vi "gums_measureLoopV2.vi"(0 "File Name":path=path "D:/users/test.dat", 1 "SaveDataQuery":bool=TRUE, 2 "Gain Cluster 2":T3={"Vsd"="Gate", "I 2probe 2"="Gate", "Vxy"="Gate", "Vxx"="Gate", "I leak BG"="Gate", "I leak TG"="Gate", "I Gain 1"=1000000.0, "V Gain 1"=1.0, "conversion factor BG"=1.0, "Vin / Vout 1"=1.0, "V Gain 2"=1.0, "Vin / Vout 2"=1.0, "V Gain 3"=1.0, "Vin / Vout 3"=1.0, "I Gain 2"=1000000.0, "I Gain 3"=1000000.0, "V BG"="Gate", "V TG"="Gate", "conversion factor TG"=1.0, "Vin / Vout 4"=1.0, "Vin / Vout 5"=1.0, "Manual Gain 1"=1.0, "Manual Gain 2"=1.0, "Manual Gain 3"=1.0} {"conversion factor TG" items=["1 V/V"=1.0, "4 V/V"=4.0, "15 V/V"=15.0, "30 V/V"=30.0, "45 V/V"=45.0]; "I Gain 3" items=["1"=1.0, "10"=10.0, "100"=100.0, "1K"=1000.0, "10K"=10000.0, "100K"=100000.0, "1M"=1000000.0, "10M"=10000000.0, "100M"=100000000.0, "1G"=1000000000.0]; "I Gain 2" items=["1"=1.0, "10"=10.0, "100"=100.0, "1K"=1000.0, "10K"=10000.0, "100K"=100000.0, "1M"=1000000.0, "10M"=10000000.0, "100M"=100000000.0, "1G"=1000000000.0]; "V Gain 3" items=["1"=1.0, "10"=10.0, "100"=100.0, "1K"=1000.0, "10K"=10000.0]; "V Gain 2" items=["1"=1.0, "10"=10.0, "100"=100.0, "1K"=1000.0, "10K"=10000.0]; "conversion factor BG" items=["1 V/V"=1.0, "4 V/V"=4.0, "15 V/V"=15.0, "30 V/V"=30.0, "45 V/V"=45.0]; "V Gain 1" items=["1"=1.0, "10"=10.0, "100"=100.0, "1K"=1000.0, "10K"=10000.0]; "I Gain 1" items=["1"=1.0, "10"=10.0, "100"=100.0, "1K"=1000.0, "10K"=10000.0, "100K"=100000.0, "1M"=1000000.0, "10M"=10000000.0, "100M"=100000000.0, "1G"=1000000000.0]}, 3 "Refresh Rate [ms]":i32=1000 min=0, 4 "Device Cluster":T4={"K2400 1"="", "K2400_1"=FALSE, "K2400 2"="", "K2400_2"=FALSE, "Lockin1"="", "Lockin1 present"=FALSE, "Lockin2"="", "Lockin2 present"=FALSE, "TIC"="", "Tcontrol"="OFF", "DAC"="", "DAC present"=FALSE, "Bfield query"=FALSE, "Wvlen query"=FALSE, "ITC signal"={"ITC"=0, "Signal"=enum."Sensor 1"}, "DMMX"=[["DMM1", ""]]}) -> ()   [LabVIEW 2011]
uses:
  gumLV8p2/D/Labviewsoft/transport/GUMS/Kelvinox drivers/ITCAPPS - Copie.LLB/ITCSignal.ctl
  gumLV8p2/D/Labviewsoft/transport/GUMS/Kelvinox drivers/ITCAPPS - Copie.LLB/ITCSignals.ctl
  gumLV8p2/D/Labviewsoft/transport/GUMS/Kelvinox drivers/BUSGEN.LLB/OxfordAddress.ctl
  stopButton.vi
  DAC/DACreadglobal.vi
  Tglobalvar.vi
  monochromatorcontrol/perHandlemonochromator.vi
  users/nicolas/PHySpec-SDK-1.0.0/Labview-example/libPhyspec/libPhyspec.lvlib
panel:
  out "refnum raw":refnum<file>
  out "DMM all (V)":dbl[](array[numeric])
  out "DMM Array":dbl[][](array[numeric])
  out "DMMX":string[][](array[string])
  out "DAC 2 V [V]":dbl=1916.0
  out "DAC 2 array":dbl[](array[numeric])
  out "Formula4Array":dbl[](array[numeric]) format="%.2f"
  out "Formula3Array":dbl[](array[numeric]) format="%.2f"
  out "Formula2Array":dbl[](array[numeric]) format="%.2f"
  in  "Formula 4":string
  in  "Formula 3":string
  in  "Formula 2":string
  out "Formula1Array":dbl[](array[numeric]) format="%.2f"
  in  "Formula 1":string
  out "Rxy Array":dbl[](array[numeric])
  out "ITC signal":T1={"ITC"=0, "Signal"=enum."Sensor 1"}
  in  "Fig3 Y scale 2":string(combo)="0"
  in  "Y-Axis 4":string(combo)="Gate"
  in  "X-Axis 4":string(combo)="Gate"
  out "Isd 4":cluster{"Bg":dbl[], "V_4probe":dbl[]}(graph)
  in  "Fig3 Y scale":string(combo)="0"
  in  "Y-Axis 3":string(combo)="Gate"
  in  "X-Axis 3":string(combo)="Gate"
  in  "Fig1 Y scale":string(combo)="0"
  in  "Fig2 Y scale":string(combo)="0"
  out "Fig 2":cluster{"Bg":dbl[], "V_4probe":dbl[]}(graph)
  in  "Y-Axis 1":string(combo)="Gate"
  in  "X-Axis 1":string(combo)="Gate"
  out "R4probe array":dbl[](array[numeric])
  out "R2probe array":dbl[](array[numeric])
  out "Itg array":dbl[](array[numeric])
  out "Ibg array":dbl[](array[numeric])
  out "Vxy array":dbl[](array[numeric])
  out "Vxx array":dbl[](array[numeric])
  out "Isd array":dbl[](array[numeric])
  out "Vsd array":dbl[](array[numeric])
  out "Vtg array":dbl[](array[numeric])
  out "Vbg array":dbl[](array[numeric])
  out "R 4probe [kOhm]":dbl=1916.0
  out "V_topgate [V]":dbl=1916.0
  out "V_backgate [V]":dbl=1916.0
  out "Vxy [V]":dbl=1916.0
  out "Vxx [V]":dbl=1916.0
  out "R 2probe [kOhm]":dbl=1916.0
  out "I Leak TG[nA]":dbl=1916.0
  out "I Leak BG [nA]":dbl=1916.0
  out "I 2probe [nA]":dbl=1916.0
  out "Vsd [V]":dbl=1916.0
  out "signal cluster":T5
  out "SetIntr Cluster":cluster{dbl, dbl, dbl, dbl, dbl, dbl, dbl}
  in  "Sensitivity Lockin2":T6(ring)
  in  "Sensitivity Lockin1":T6(ring)
  out "Wavelength array":dbl[](array[numeric])
  out "Wavelength [nm]":dbl=1916.0
  out "Wvlen query":bool
  out "refnum data":refnum<file>
  in  "Y-Axis 2":string(combo)="Gate"
  in  "X-Axis 2":string(combo)="Gate"
  out "I K2400 01":dbl[](array[numeric])
  out "I K2400 02":dbl[](array[numeric])
  out "DAC 4 array":dbl[](array[numeric])
  out "DAC 3 array":dbl[](array[numeric])
  out "B":dbl[](array[numeric])
  out "Lockin2 X":dbl[](array[numeric])
  out "Lockin2 Y":dbl[](array[numeric])
  out "Lockin1 X":dbl[](array[numeric])
  out "B [T]":dbl=1916.0
  out "T [K]":dbl=1916.0
  out "Bfield query":bool
  out "I K2400_2 [A]":dbl=1916.0
  out "Lockin2 Y [V]":dbl=1916.0
  out "Lockin2 X [V]":dbl=1916.0
  out "DAC 4 V [V]":dbl=1916.0
  out "DAC 3 V [V]":dbl=1916.0
  out "I K2400_1 [A]":dbl=1916.0
  out "Lockin1 Y [V]":dbl=1916.0
  out "Lockin1 X [V]":dbl=1916.0
  out "Lockin1 Ampl [V]":dbl=1916.0
  out "K2400 1 [V]":dbl=1916.0
  out "K2400 2 [V]":dbl=1916.0
  out "DAC 1 V [V]":dbl=1916.0
  out "DAC present":bool
  out "K2400_2":bool
  out "K2400 2":refnum<visa-resource-name>="GPIB0::11::INSTR"
  out "DAC":refnum<visa-resource-name>="GPIB0::11::INSTR"
  out "Tcontrol":string
  out "Lockin2 present":bool
  out "Lockin1 present":bool
  out "K2400_1":bool
  out "TIC":refnum<visa-resource-name>="GPIB0::11::INSTR"
  out "Lockin2":refnum<visa-resource-name>="GPIB0::11::INSTR"
  out "Lockin1":refnum<visa-resource-name>="GPIB0::11::INSTR"
  out "K2400 1":refnum<visa-resource-name>="GPIB0::11::INSTR"
  out "Isd":cluster{"Bg":dbl[], "V_4probe":dbl[]}(graph)
  out "Isd 3":cluster{"Bg":dbl[], "V_4probe":dbl[]}(graph)
  out "stopMainLoop":bool
  out "V K2400_01 array":dbl[](array[numeric])
  out "Lockin1 Y":dbl[](array[numeric])
  out "DAC 1 array":dbl[](array[numeric])
  out "V K2400_02 array":dbl[](array[numeric])
  out "T":dbl[](array[numeric])
  out "Time":dbl[](array[numeric])
  out "Time [s]":dbl=1916.0
  in  "stop":bool
  # "Current run values"
  # "Magnetic Field"
  # "Wavelength"
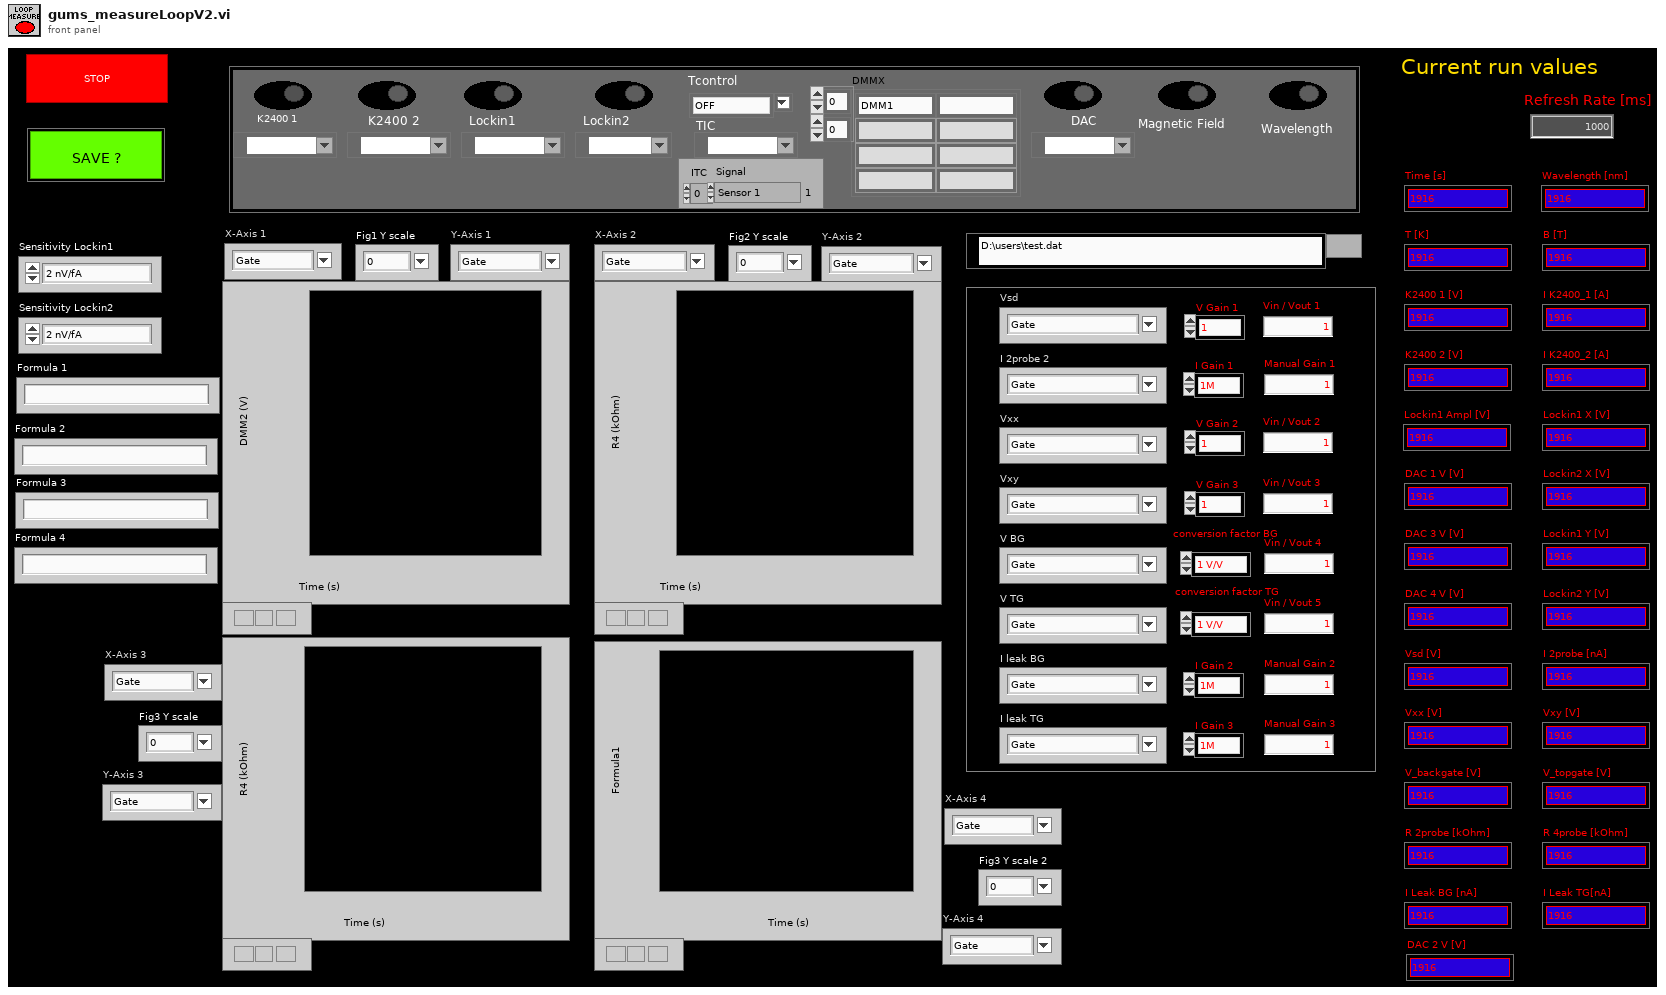
[diagram p1: front panel]
types:
  T1 = typedef "ITCSignal.ctl" = cluster{"ITC":u16, "Signal":T2}
  T2 = typedef "ITCSignals.ctl" = enum16{"Setpoint", "Sensor 1", "Sensor 2", "Sensor 3", "Needle Valve %", "Heater %"}
  T3 = cluster{"Vsd":string, "I 2probe 2":string, "Vxy":string, "Vxx":string, "I leak BG":string, "I leak TG":string, "I Gain 1":dbl, "V Gain 1":dbl, "conversion factor BG":dbl, "Vin / Vout 1":dbl, "V Gain 2":dbl, "Vin / Vout 2":dbl, "V Gain 3":dbl, "Vin / Vout 3":dbl, "I Gain 2":dbl, "I Gain 3":dbl, "V BG":string, "V TG":string, "conversion factor TG":dbl, "Vin / Vout 4":dbl, "Vin / Vout 5":dbl, "Manual Gain 1":dbl, "Manual Gain 2":dbl, "Manual Gain 3":dbl}
  T4 = cluster{"K2400 1":refnum<visa-resource-name>, "K2400_1":bool, "K2400 2":refnum<visa-resource-name>, "K2400_2":bool, "Lockin1":refnum<visa-resource-name>, "Lockin1 present":bool, "Lockin2":refnum<visa-resource-name>, "Lockin2 present":bool, "TIC":refnum<visa-resource-name>, "Tcontrol":string, "DAC":refnum<visa-resource-name>, "DAC present":bool, "Bfield query":bool, "Wvlen query":bool, "ITC signal":T1, "DMMX":string[][]}
  T5 = cluster{"Output X":dbl, "Output X":dbl, dbl, dbl, "DMM array all (V)":dbl[]}
  T6 = enum16{"2 nV/fA", "5 nV/fA", "10 nV/fA", "20 nV/fA", "50 nV/fA", "100 nV/fA", "200 nV/fA", "500 nV/fA", "1 uV/pA", "2 uV/pA", "5 uV/pA", "10 uV/pA", "20 uV/pA", "50 uV/pA", "100 uV/pA", "200 uV/pA", "500 uV/pA", "1 mV/nA", "2 mV/nA", "5 mV/nA", "10 mV/nA", "20 mV/nA", "50 mV/nA", "100 mV/nA", "200 mV/nA", "500 mV/nA", "1 V/uA"}
  T7 = typedef "OxfordAddress.ctl" = cluster{"Com Port":i32, "ISOBUS Address":i32, "GPIB Address":i16, "Communication":enum16{"RS232", "ISOBUS", "GPIB", "Gateway"}}
  T8 = enum16{"open", "replace", "create", "open or create", "replace or create", "replace or create with confirmation"}
  T9 = cluster{"Output X":dbl, "Output X":dbl, "I K2400_1 [A]":dbl, "I K2400_2 [A]":dbl, dbl[]}
  T10 = cluster{"Formula4Array":dbl[], "Formula4Array":dbl[]}
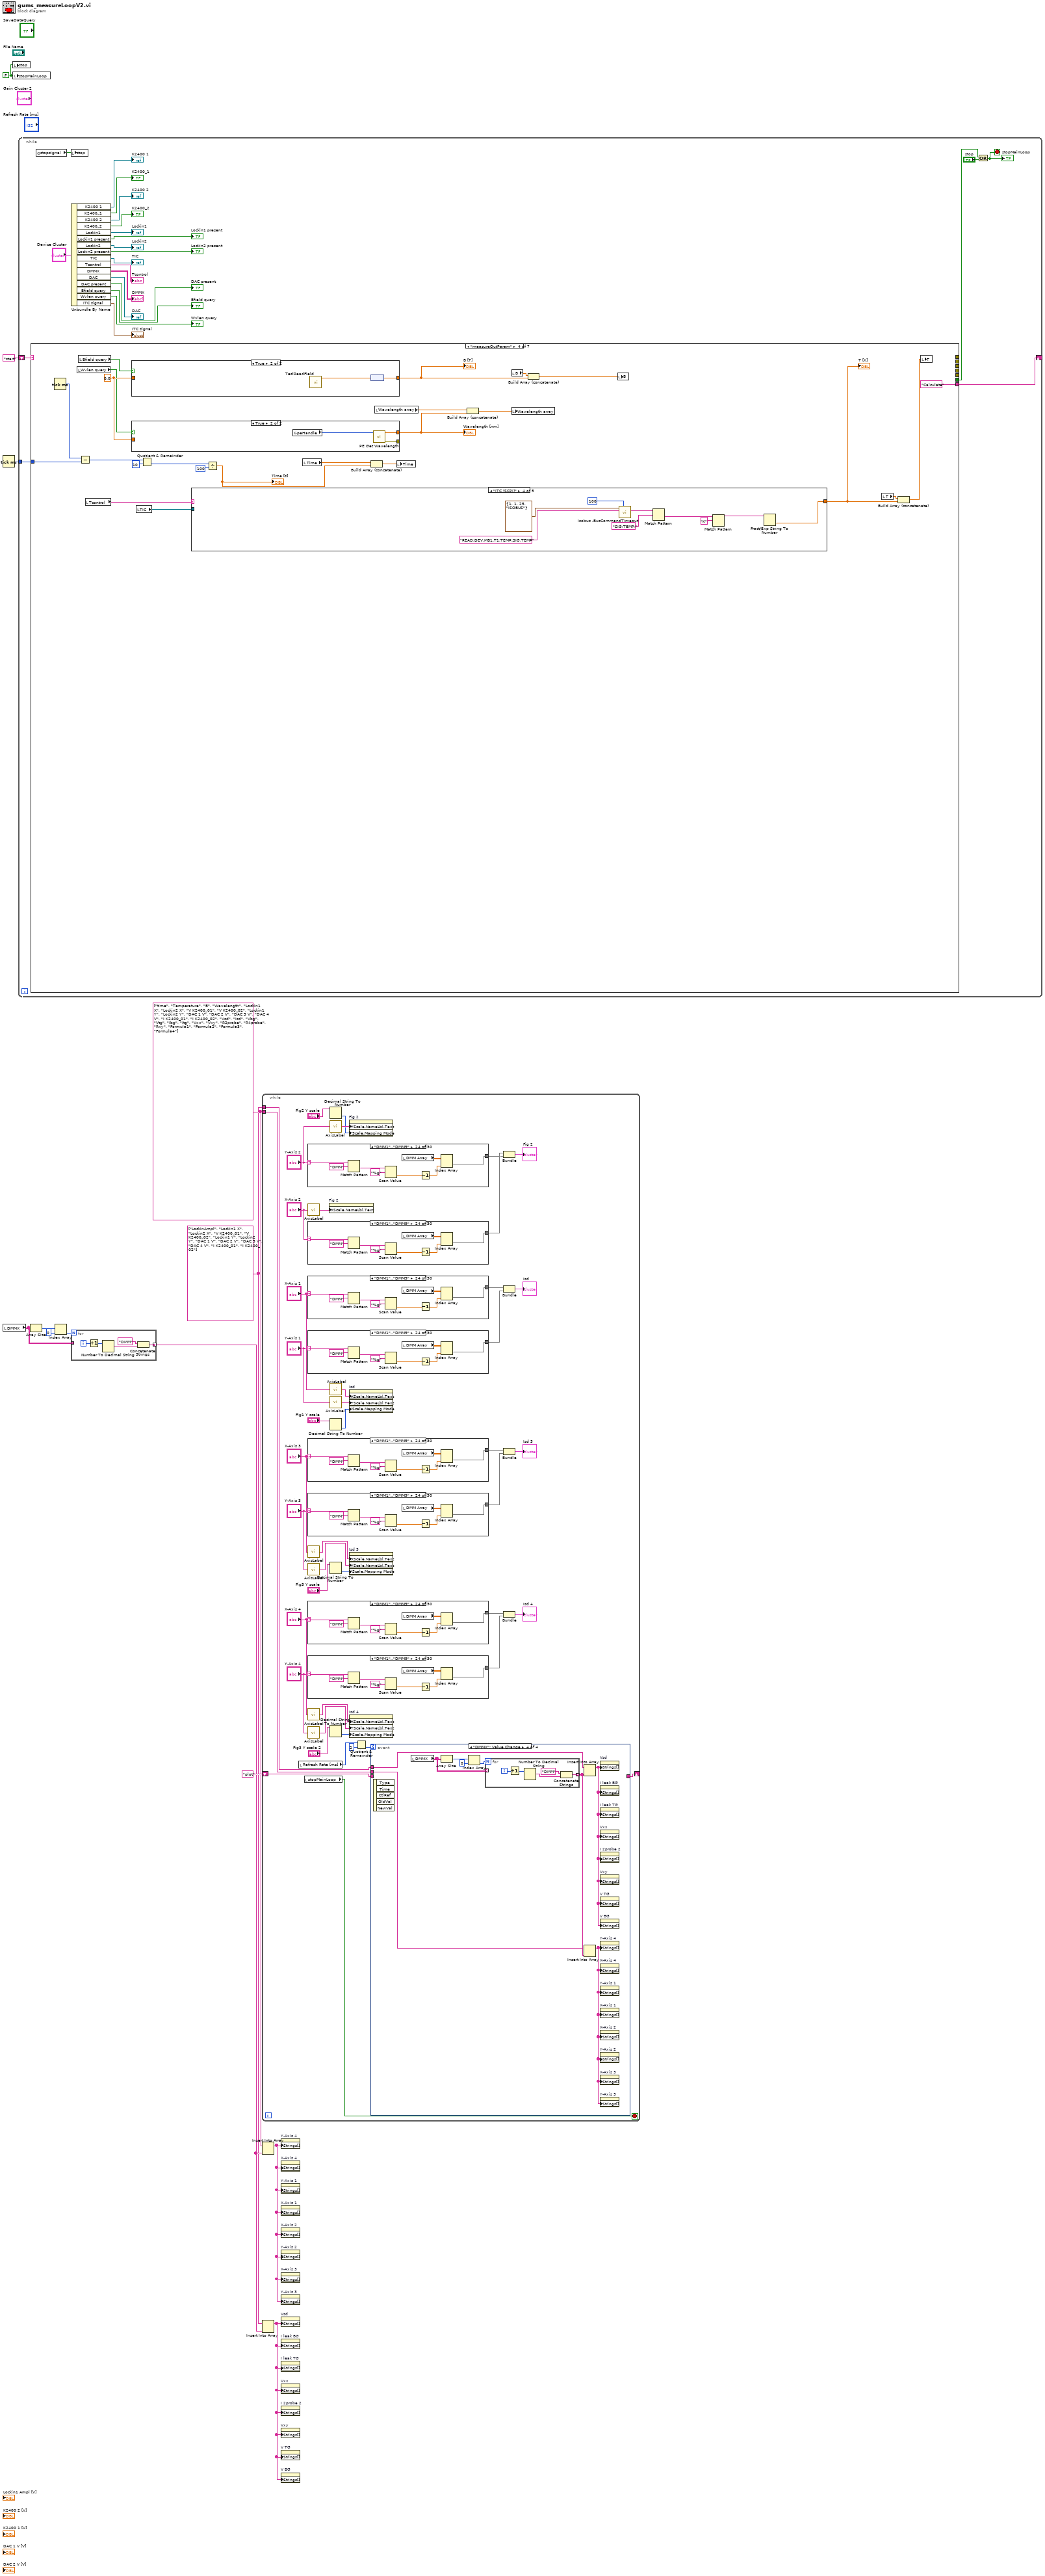
[diagram p0: block diagram]
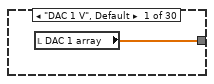
[diagram p2: hidden frame]
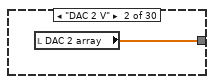
[diagram p3: hidden frame]
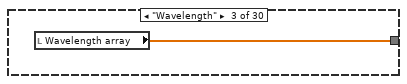
[diagram p4: hidden frame]
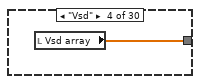
[diagram p5: hidden frame]
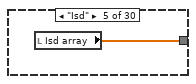
[diagram p6: hidden frame]
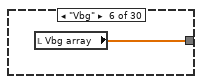
[diagram p7: hidden frame]
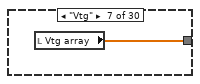
[diagram p8: hidden frame]
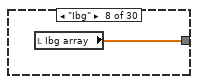
[diagram p9: hidden frame]
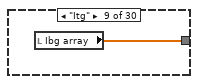
[diagram p10: hidden frame]
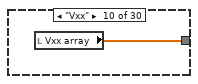
[diagram p11: hidden frame]
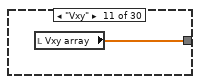
[diagram p12: hidden frame]
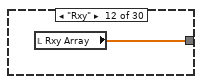
[diagram p13: hidden frame]
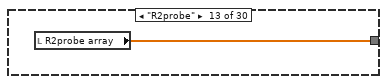
[diagram p14: hidden frame]
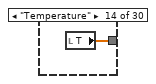
[diagram p15: hidden frame]
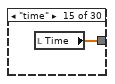
[diagram p16: hidden frame]
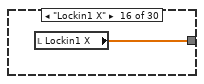
[diagram p17: hidden frame]
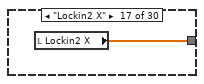
[diagram p18: hidden frame]
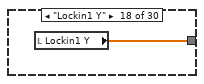
[diagram p19: hidden frame]
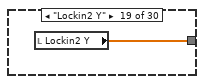
[diagram p20: hidden frame]
diagram:
  w2 = string[] ["time", "Temperature", "B", "Wavelength", "Lockin1 X", "Lockin2 X", "V K2400_01", "V K2400_02", "Lockin1 Y", "Lockin2 Y", "DAC 1 V", "DAC 2 V", "DAC 3 V", "DAC 4 V", "I K2400_01", "I K2400_02", "Vsd", "Isd", "Vbg", "Vtg", "Ibg", "Itg", "Vxx", "Vxy", "R2probe", "R4probe", "Rxy", "Formula1", "Formula2", "Formula3", "Formula4"] ("Axis select")
  w1 = string[] ["LockinAmpl", "Lockin1 X", "Lockin2 X", "V K2400_01", "V K2400_02", "Lockin1 Y", "Lockin2 Y", "DAC 1 V", "DAC 2 V", "DAC 3 V", "DAC 4 V", "I K2400_01", "I K2400_02"] ("Strings []")
  w11 = FALSE ("stop")
  n1 = Tick Count (ms)() -> (millisecond timer value=w12:u32)
  n2 = local read "DMMX"() -> (w7:string[][])
  n3 = local write "stop"(w11) -> ()
  n4 = local write "stopMainLoop"(w11) -> ()
  n5 = while {
    shift-right: [w36] -> _
    shift-left: "start" -> [w37]
    tunnel: w12 -> [w33]
    stop <- w32 stop-if-true
    n6 = case shown="\"measureOutParam\"" w37 {
      tunnel: ["measureSetInstruments" "measureSignal" "measureOutParam" "Calculate" "measureSetInstruments" "writeFile" ""] -> w36
      tunnel: [_ _ _ _ _ _ TRUE ("x")] -> w34
      tunnel: w33 -> [_ _ _ w300 _ _ _]
      tunnel: [_ _ _ _ w331 _ _] -> _
      tunnel: [_ _ _ _ _ w445 _] -> _
      tunnel: [_ _ _ _ _ w435 _] -> _
      tunnel: [_ _ _ _ _ w434 _] -> _
      tunnel: [_ _ _ _ _ w433 _] -> _
      frame "start", Default {
        w42 = enum16{"start", "end", "current"}."end" ("from (0:start)")
        w47 = T8."open or create" ("operation (0:open)")
        w74 = 0 ("dimension size")
        w81 = "\t"
        w88 = "\t"
        w96 = "\t"
        w57 = "\t"
        w100 = "\t"
        w97 = "\t"
        w107 = "\t"
        # "Time\nT\nB\nWavelength\nDAC1\nDAC2\nDAC3\nDAC4\nV K2400_01\nV K2400_02\nLockin V\nLK 1 X\nLK 1 Y\nLK2 X\nLK2 Y\nDMMX\nI K2400_01\nI K2400_02\n\nTime\nT\nB\nWavelength\nVsd\nVbgate\nVtopgate\nI2probe\nIleak bg\nIleak tg\nVxx\nVxy\nR2probe\nR4probe"
        n7 = Get Date/Time In Seconds() -> (seconds since 1Jan1904=w118:timestamp)
        n8 = Initialize Array(w74, w74, w74) -> (→"DMM Array":i32[][])
        n9 = Initialize Array(0) -> (→"Time" →"T" →"DAC 1 array" →"V K2400_01 array" →"V K2400_02 array" →"Lockin1 Y" →"Lockin1 X" →"Lockin2 Y" →"Lockin2 X" →"B" →"DAC 3 array" →"DAC 4 array" →"I K2400 02" →"I K2400 01" →"Wavelength array" →"Vbg array" →"Vtg array" →"Vsd array" →"Isd array" →"Vxx array" →"Vxy array" →"Ibg array" →"Itg array" →"R2probe array" →"R4probe array" →"Rxy Array" →"DAC 2 array":i32[])  [unwired: 1 out]
        n10 = local read "File Name"() -> (w67:path)
        n11 = local read "DMMX"() -> (w50:string[][])
        n12 = Get Date/Time String(date format (0)=1, seconds (now)=w118) -> (date string=w115:string, time string=w116:string)  [unwired: 1 out]
        n13 = Array Size(array=w50) -> (size(s)=w53:i32[])
        n14 = Strip Path(path=w67) -> (stripped path=w72:path, name=w71:string)
        n15 = Concatenate Strings("I K2400_01 [A]" ("string"), w97, "I K2400_02 [A]" ("string"), w97) -> (w51:string)
        n16 = Open/Create/Replace File(file path (use dialog)=w67, prompt="Enter data filename", operation (0:open)=w47) -> (refnum out=w46:refnum<file>, error out=w45:errorcluster)  [unwired: 1 in, 3 out]
        n17 = Concatenate Strings(w116, "\t", w115, "\r\n") -> (w61:string)
        n18 = Index Array(array=w53, index=0) -> (element=w52:i32)
        n19 = for {
          N: w52 -> [_]
          tunnel: [w124] -> w49 mode=indexing
          i -> [w127]
          n20 = Increment(x=w127) -> (x+1=w125:i32)
          n21 = Number To Decimal String(number=w125) -> (decimal integer string=w126:string)  [unwired: 1 in]
          n22 = Concatenate Strings("DMM", w126, " [V]" ("string"), "\t") -> (w124:string)
        }
        n23 = Concatenate Strings("Vxx [V]" ("string"), w81, "Vxy [V]" ("string"), w81, "R2probe [kOhm]" ("string"), w81, "R4probe [kOhm]" ("string")) -> (w80:string)
        n24 = Concatenate Strings("Vsd [V]" ("string"), w96, "Vbg [V]" ("string"), w96, "Vtg [V]" ("string"), w96) -> (w92:string)
        n25 = Concatenate Strings("I 2probe [nA]" ("string"), w88, "Ileak bg [nA]" ("string"), w88, "Ileak tg [nA]" ("string"), w88) -> (w86:string)
        n26 = Concatenate Strings("Time [s]", w107, "T [K]" ("chaîne"), w107, "B [T]" ("chaîne"), w107, "Wavelength [nm]" ("chaîne"), w107) -> (w58:string)
        n27 = Search and Replace String(input string=w71, search string=".dat", replace string="_raw.dat" ("replace string (\"\")")) -> (result string=w68:string)  [unwired: 5 in, 3 out]
        n28 = Set File Position(refnum=w46, from (0:start)=w42, error in=w45) -> (refnum out=w43:refnum<file>, error out=w44:errorcluster)  [unwired: 1 in]
        n29 = Build Path(base path=w72, name or relative path=w68) -> (appended path=w66:path)
        n30 = Concatenate Strings(w61, w58, w92, w86, w80, "\r\n") -> (w112:string)
        n31 = Write to Text File(file (use dialog)=w43, text=w112, error in=w44) -> (refnum out=→"refnum data":refnum<file>, error out=w65:errorcluster)  [unwired: 2 out]
        n32 = Concatenate Strings("DAC 1 [V]" ("string"), w57, "DAC 2 [V]" ("string"), w57, "DAC 3 [V]" ("string"), w57, "DAC 4 [V]" ("string"), w57, "K2400_01 [V]" ("string"), w57, "K2400_02 [V]" ("string"), w57, "Lockin V [V]" ("string"), w57) -> (w59:string)
        n33 = Concatenate Strings("Lockin1 X [V]" ("string"), w100, "Lockin1 Y [V]" ("string"), w100, "Lockin2 X [V]" ("string"), w100, "Lockin2 Y [V]" ("string"), w100) -> (w60:string)
        n34 = Open/Create/Replace File(file path (use dialog)=w66, error in=w65, operation (0:open)=w47) -> (refnum out=w39:refnum<file>, error out=w41:errorcluster)  [unwired: 1 in, 3 out]
        n35 = Concatenate Strings(w61, w58, w59, w60, w49, w51, "\r\n") -> (w48:string)
        n36 = Set File Position(refnum=w39, from (0:start)=w42, error in=w41) -> (refnum out=w38:refnum<file>, error out=w40:errorcluster)  [unwired: 1 in]
        n37 = Write to Text File(file (use dialog)=w38, text=w48, error in=w40) -> (refnum out=→"refnum raw":refnum<file>, error out=w63:errorcluster)  [unwired: 2 out]
        n38 = case shown="No Error" w63 {
          frame No Error {
          }
          frame Error {
          }
        }
      }
      frame "measureSetInstruments" {
        w144 = errorcluster {"status"=FALSE, "code"=0, "source"=""} ("error in (no error)")
        w140 = 0.0
        # "DAC 1\nK2400 1\nK2400 2\nLockin\nDAC 2\nDAC 3\nDAC 4"
        n39 = local read "K2400_1"() -> (w161:bool)
        n40 = local read "K2400_2"() -> (w160:bool)
        n41 = local read "K2400 1"() -> (w153:refnum<visa-resource-name>)
        n42 = local read "K2400 2"() -> (w152:refnum<visa-resource-name>)
        n43 = local read "Lockin1 present"() -> (w150:bool)
        n44 = local read "Lockin1"() -> (w151:refnum<visa-resource-name>)
        n45 = case shown="True" w161 {
          tunnel: [w203 w208] -> w148
          tunnel: w140 -> [w203 _]
          tunnel: w153 -> [_ w207]
          tunnel: w144 -> [_ _]
          tunnel: [w203 w204] -> w143
          frame False {
          }
          frame True {
            n46 = call "K2400_write&read.vi"("Command"="READ?", "VISA Resource Name"=w207) -> ("error out"=w206:errorcluster, "Read"=w212:string)  [unwired: 1 in]
            n47 = case shown="No Error" w206 {
              frame No Error {
              }
              frame Error {
              }
            }
            n48 = Match Pattern(string=w212, regular expression=",") -> (before substring=w209:string, after substring=w205:string)  [unwired: 3 out]
            n49 = Fract/Exp String To Number(string=w209) -> (number=w208:dbl)  [unwired: 4 out]
            n50 = Fract/Exp String To Number(string=w205) -> (number=w204:dbl)  [unwired: 4 out]
          }
        }
        "I K2400_1 [A]" <- w143
        n51 = case shown="True" w160 {
          tunnel: [w192 w198] -> w146
          tunnel: w140 -> [w192 _]
          tunnel: w152 -> [_ w197]
          tunnel: w144 -> [_ w196]
          tunnel: [w192 w193] -> w142
          frame False {
          }
          frame True {
            n52 = call "K2400_write&read.vi"("error in (no error)"=w196, "Command"="READ?", "VISA Resource Name"=w197) -> ("error out"=w195:errorcluster, "Read"=w202:string)
            n53 = case shown="No Error" w195 {
              frame No Error {
              }
              frame Error {
              }
            }
            n54 = Match Pattern(string=w202, regular expression=",") -> (before substring=w199:string, after substring=w194:string)  [unwired: 3 out]
            n55 = Fract/Exp String To Number(string=w199) -> (number=w198:dbl)  [unwired: 4 out]
            n56 = Fract/Exp String To Number(string=w194) -> (number=w193:dbl)  [unwired: 4 out]
          }
        }
        "I K2400_2 [A]" <- w142
        n57 = global read "DACreadglobal.vi" "DAC read global (mV)"() -> (w136:dbl[])
        n58 = local read "DAC present"() -> (w137:bool)
        n59 = case shown="True" w150 {
          tunnel: [w163 w165] -> w147
          tunnel: w140 -> [w163 _]
          tunnel: w151 -> [_ w164]
          frame False {
          }
          frame True {
            n60 = VISA Write(VISA resource name=w164, write buffer="SLVL? " ("chaîne")) -> (VISA resource name out=w169:refnum<visa-resource-name>, error out=w168:errorcluster)  [unwired: 1 in, 1 out]
            n61 = VISA Read(VISA resource name=w169, byte count=u32 1024, error in (no error)=w168) -> (read buffer=w166:string)  [unwired: 3 out]
            n62 = Fract/Exp String To Number(string=w166) -> (number=w165:dbl)  [unwired: 4 out]
          }
        }
        n63 = local read "DAC"() -> (w141:refnum<visa-resource-name>)
        n64 = case shown="True" w137 {
          selector: w137 -> [w173 w189]
          tunnel: [w171 w190] -> w149
          tunnel: w140 -> [w171 _]
          tunnel: w141 -> [_ _]
          tunnel: [w173 w189] -> _
          tunnel: w136 -> [w172 w176]
          tunnel: [w172 w176] -> _
          tunnel: [w171 w183] -> w135
          tunnel: [w171 w175] -> w130
          tunnel: [w171 w174] -> w129
          frame False {
          }
          frame True {
            # "dac 4"
            # "dac 3"
            n65 = Index Array(array=w176, index=2) -> (element=w182:dbl)
            n66 = Index Array(array=w176, index=3) -> (element=w179:dbl)
            n67 = Index Array(array=w176, index=0) -> (element=w187:dbl)
            n68 = Index Array(array=w176, index=1) -> (element=w186:dbl)
            n69 = Divide(x=w182, y=1000.0) -> (x/y=w175:dbl)
            n70 = Divide(x=w179, y=1000.0) -> (x/y=w174:dbl)
            n71 = Divide(x=w187, y=1000.0) -> (x/y=w190:dbl)
            n72 = Divide(x=w186, y=1000.0) -> (x/y=w183:dbl)
          }
        }
        "DAC 3 V [V]" <- w130
        "DAC 4 V [V]" <- w129
        n73 = local read "DAC 1 array"() -> (w159:dbl[])
        n74 = local read "DAC 3 array"() -> (w134:dbl[])
        n75 = local read "DAC 4 array"() -> (w132:dbl[])
        n76 = local read "DAC 2 array"() -> (w139:dbl[])
        n77 = local read "V K2400_01 array"() -> (w156:dbl[])
        n78 = local read "V K2400_02 array"() -> (w157:dbl[])
        n79 = local write "DAC 2 V [V]"(w135) -> ()
        n80 = local write "Lockin1 Ampl [V]"(w147) -> ()
        n81 = local write "DAC 1 V [V]"(w149) -> ()
        n82 = Build Array (concatenate)(w159, w149) -> (w158:dbl[])
        n83 = Build Array (concatenate)(w134, w130) -> (w133:dbl[])
        n84 = Build Array (concatenate)(w132, w129) -> (w131:dbl[])
        n85 = Build Array (concatenate)(w139, w135) -> (w138:dbl[])
        n86 = local write "DAC 1 array"(w158) -> ()
        n87 = local write "DAC 3 array"(w133) -> ()
        n88 = local write "DAC 4 array"(w131) -> ()
        n89 = local write "DAC 2 array"(w138) -> ()
        n90 = local write "K2400 1 [V]"(w148) -> ()
        n91 = local write "K2400 2 [V]"(w146) -> ()
        n92 = Bundle(w149, w148, w146, w147, w135, w130, w129) -> (→"SetIntr Cluster":cluster{dbl, dbl, dbl, dbl, dbl, dbl, dbl})  [unwired: 1 in]
        n93 = Build Array (concatenate)(w156, w148) -> (w154:dbl[])
        n94 = Build Array (concatenate)(w157, w146) -> (w155:dbl[])
        n95 = local write "V K2400_01 array"(w154) -> ()
        n96 = local write "V K2400_02 array"(w155) -> ()
      }
      frame "measureSignal" {
        w244 = 0.0
        # "lockin1 X\nLockin2 X\nI K2400 01\nI K2400 02\nDMMxxx"
        n97 = local read "K2400_1"() -> (w251:bool)
        n98 = local read "K2400 1"() -> (w252:refnum<visa-resource-name>)
        n99 = local read "DMMX"() -> (w218:string[][])
        n100 = local read "Lockin1 present"() -> (w249:bool)
        n101 = local read "Lockin1"() -> (w250:refnum<visa-resource-name>)
        n102 = Array Size(array=w218) -> (size(s)=w220:i32[])
        n103 = case shown="False" w251 {
          tunnel: [w271 w272] -> w223
          tunnel: w252 -> [_ _]
          tunnel: w244 -> [w271 _]
          tunnel: "READ?" -> [w270 w273]
          tunnel: [w270 w273] -> w226
          frame False {
          }
          frame True {
            n104 = local read "I K2400_1 [A]"() -> (w272:dbl)
          }
        }
        n105 = Index Array(array=w220, index=0) -> (element=w217:i32)
        n106 = case shown="True" w249 {
          tunnel: w250 -> [_ w280]
          tunnel: [w274 w279] -> w213
          tunnel: [w274 w278] -> w232
          tunnel: w244 -> [w274 w276]
          tunnel: [w275 w277] -> w228
          tunnel: "1,4" ("Variable") -> [w275 w277]
          tunnel: [w274 w276] -> w225
          frame False {
          }
          frame True {
            n107 = call "Lockin_SR830_readXY.vi"("Variable"=w277, "VISA Resource Name"=w280) -> ("Output Y"=w278:dbl, "Output X"=w279:dbl)
          }
        }
        "Lockin1 X [V]" <- w213
        "Lockin1 Y [V]" <- w232
        n108 = for {
          N: w217 -> [_]
          tunnel: w218 -> [w262] mode=indexing
          tunnel: [w256] -> _ mode=indexing
          tunnel: [w255] -> w214 mode=indexing
          n109 = Index Array(array=w262, index=1) -> (element=w258:string)
          n110 = Concatenate Strings("GPIB0::" ("string"), w258) -> (w257:string)
          n111 = Type Cast(type=refnum<visa-resource-name> refnum ("VISA resource name"), x=w257) -> (*(type *) &x=w256:refnum<visa-resource-name>)
          n112 = call "AGILENT34401a_read.vi"("VISA Resource Name in"=w256) -> ("Voltage output"=w255:dbl, "error out"=w254:errorcluster)  [unwired: 1 out]
          n113 = case shown="No Error" w254 {
            frame No Error {
            }
            frame Error {
            }
          }
        }
        "DMM all (V)" <- w214
        n114 = local read "I K2400 01"() -> (w243:dbl[])
        n115 = local read "K2400_2"() -> (w245:bool)
        n116 = local read "K2400 2"() -> (w246:refnum<visa-resource-name>)
        n117 = local read "Lockin2 present"() -> (w247:bool)
        n118 = local read "Lockin1 X"() -> (w236:dbl[])
        n119 = local read "Lockin1 Y"() -> (w233:dbl[])
        n120 = local read "Lockin2"() -> (w248:refnum<visa-resource-name>)
        n121 = case shown="False" w245 {
          tunnel: [w263 w264] -> w221
          tunnel: w246 -> [_ _]
          tunnel: w244 -> [w263 _]
          tunnel: w226 -> [_ _]
          frame False {
          }
          frame True {
            n122 = local read "I K2400_2 [A]"() -> (w264:dbl)
          }
        }
        n123 = Build Array (concatenate)(w243, w223) -> (w242:dbl[])
        n124 = case shown="True" w247 {
          tunnel: w248 -> [_ w269]
          tunnel: [w265 w268] -> w224
          tunnel: [w265 w267] -> w238
          tunnel: w225 -> [w265 _]
          tunnel: w228 -> [_ w266]
          frame False {
          }
          frame True {
            n125 = call "Lockin_SR830_readXY.vi"("Variable"=w266, "VISA Resource Name"=w269) -> ("Output Y"=w267:dbl, "Output X"=w268:dbl)
          }
        }
        "Lockin2 X [V]" <- w224
        "Lockin2 Y [V]" <- w238
        n126 = local write "I K2400 01"(w242) -> ()
        n127 = Build Array (concatenate)(w236, w213) -> (w235:dbl[])
        n128 = Build Array (concatenate)(w233, w232) -> (w234:dbl[])
        n129 = local write "Lockin1 X"(w235) -> ()
        n130 = local write "Lockin1 Y"(w234) -> ()
        n131 = local read "I K2400 02"() -> (w230:dbl[])
        n132 = local read "Lockin2 X"() -> (w241:dbl[])
        n133 = local read "Lockin2 Y"() -> (w239:dbl[])
        n134 = Build Array (concatenate)(w230, w221) -> (w231:dbl[])
        n135 = local read "DMM Array"() -> (w216:dbl[][])
        n136 = local write "I K2400 02"(w231) -> ()
        n137 = Build Array (concatenate)(w241, w224) -> (w240:dbl[])
        n138 = Build Array (concatenate)(w239, w238) -> (w237:dbl[])
        n139 = local write "Lockin2 X"(w240) -> ()
        n140 = local write "Lockin2 Y"(w237) -> ()
        n141 = Bundle("Output X"=w213, "Output X"=w224, "I K2400_1 [A]"=w223, "I K2400_2 [A]"=w221, w214) -> (→"signal cluster":T9)  [unwired: 1 in]
        n142 = Build Array (concatenate)(w216, w214) -> (w215:dbl[][])
        n143 = local write "DMM Array"(w215) -> ()
      }
      frame "measureOutParam" {
        w288 = 0.0
        n144 = Tick Count (ms)() -> (millisecond timer value=w303:u32)
        n145 = local read "Wvlen query"() -> (w287:bool)
        n146 = local read "Bfield query"() -> (w298:bool)
        n147 = Subtract(x=w303, y=w300) -> (x-y=w301:u32)
        n148 = local read "Tcontrol"() -> (w299:string)
        n149 = case shown="True" w298 {
          tunnel: [w309 w310] -> w292
          tunnel: w288 -> [w309 _]
          frame False {
          }
          frame True {
            n150 = call "TeslReadField.vi"() -> ("Effective field"=w311:dbl[unit])  [unwired: 6 in, 1 out]
            n151 = node(w311) -> (w310:dbl)
          }
        }
        "B [T]" <- w292
        n152 = case shown="True" w287 {
          tunnel: w288 -> [w305 _]
          tunnel: [w305 w307] -> w285
          tunnel: [_ w306] -> _
          frame False {
          }
          frame True {
            n153 = global read "perHandlemonochromator.vi" "peHandle"() -> (w308:u32)
            n154 = call "PE Get Wavelength.vi"("peHandle"=w308) -> ("error out"=w306:errorcluster, "wavelength"=w307:dbl)  [unwired: 8 in, 1 out]
          }
        }
        "Wavelength [nm]" <- w285
        n155 = local read "TIC"() -> (w291:refnum<visa-resource-name>)
        n156 = Quotient & Remainder(x=w301, y=u32 10) -> (floor(x/y)=w283:u32)  [unwired: 1 out]
        n157 = case shown="\"ITC (SCPI)\"" w299 {
          tunnel: [0.0 w314 w318 w320 w329] -> w295
          tunnel: w291 -> [_ w313 _ _ _]
          frame "OFF", Default {
          }
          frame "TIC (OeLab)" {
            n158 = call "TIC_rw.vi"("write buffer"="in1.value?", "TIC 500"=w313) -> ("read buffer"=w316:string)  [unwired: 1 in, 2 out]
            n159 = Scan Value(string=w316, format string="%.3f") -> (value=w314:dbl)  [unwired: 1 in, 1 out]
          }
          frame "ITC" {
            n160 = local read "ITC signal"() -> (w319:T1)
            n161 = call "ITCGetReading.vi"("Signal"=w319) -> ("Reading"=w318:dbl)  [unwired: 6 in]
          }
          frame "ITC (SCPI)" {
            n162 = call "Isobus -BusCommandTimeout.vi"("Timeout (ms)"=u32 100, "Command"="READ:DEV:MB1.T1:TEMP:SIG:TEMP", "Address"=T7 {"Com Port"=1, "ISOBUS Address"=1, "GPIB Address"=25, "Communication"=enum."ISOBUS"}) -> ("Reply"=w325:string)  [unwired: 5 out]
            n163 = Match Pattern(string=w325, regular expression="SIG:TEMP:") -> (after substring=w323:string)  [unwired: 1 in, 3 out]
            n164 = Match Pattern(string=w323, regular expression="K") -> (before substring=w321:string)  [unwired: 1 in, 3 out]
            n165 = Fract/Exp String To Number(string=w321) -> (number=w320:dbl)  [unwired: 3 in, 1 out]
          }
          frame "GlobalVar" {
            n166 = global read "Tglobalvar.vi" "Tglobalvar"() -> (w329:dbl)
          }
        }
        "T [K]" <- w295
        n167 = Divide(x=w283, y=u32 100) -> (x/y=w281:dbl)
        "Time [s]" <- w281
        n168 = local read "Time"() -> (w289:dbl[])
        n169 = Build Array (concatenate)(w289, w281) -> (w290:dbl[])
        n170 = local read "Wavelength array"() -> (w286:dbl[])
        n171 = local write "Time"(w290) -> ()
        n172 = Build Array (concatenate)(w286, w285) -> (w284:dbl[])
        n173 = local read "B"() -> (w294:dbl[])
        n174 = local write "Wavelength array"(w284) -> ()
        n175 = Build Array (concatenate)(w294, w292) -> (w293:dbl[])
        n176 = local write "B"(w293) -> ()
        n177 = local read "T"() -> (w296:dbl[])
        n178 = Build Array (concatenate)(w296, w295) -> (w297:dbl[])
        n179 = local write "T"(w297) -> ()
      }
      frame "writeFile" {
        n180 = local read "SaveDataQuery"() -> (w330:bool)
        n181 = case shown="True" w330 {
          frame False {
          }
          frame True {
            w356 = "\t"
            w367 = "\t"
            w374 = "\t"
            w354 = "\t"
            w389 = "\t"
            w341 = "\t"
            w334 = "\r\n"
            w381 = "\t"
            # "Time\nT\nB\nWavelength\nDAC1\nDAC2\nDAC3\nDAC4\nV K2400_01\nV K2400_02\nLockin V\nLK 1 X\nLK 1 Y\nLK2 X\nLK2 Y\nDMMX\nI K2400_01\nI K2400_02\n\nTime\nT\nB\nWavelength\nVsd\nVbgate\nVtopgate\nI2probe\nIleak bg\nIleak tg\nVxx\nVxy\nR2probe\nR4probe"
            # "I K2400_01\nI K2400_02"
            # "LK 1 X\nLK 1 Y\nLK2 X\nLK2 Y"
            # "DACs\nV K2400_01\nV K2400_02\nLockin V"
            # "Time\nT\nB\nWavelength"
            # "Time\nT\nB\nDAC\nV K2400_01\nV K2400_02\nLockin V\nDMM1\nDMM2\nLK 1 X\nLK 1 Y\nLK2 X\nLK2 Y\nI K2400_01\nI K2400_02"
            n182 = local read "DMM all (V)"() -> (w338:dbl[])
            n183 = local read "Wavelength [nm]"() -> (w383:dbl)
            n184 = local read "R 2probe [kOhm]"() -> (w362:dbl)
            n185 = local read "R 4probe [kOhm]"() -> (w361:dbl)
            n186 = local read "Lockin1 Ampl [V]"() -> (w399:dbl)
            n187 = local read "V_backgate [V]"() -> (w378:dbl)
            n188 = local read "I Leak BG [nA]"() -> (w370:dbl)
            n189 = local read "V_topgate [V]"() -> (w377:dbl)
            n190 = local read "I Leak TG[nA]"() -> (w371:dbl)
            n191 = local read "Lockin1 X [V]"() -> (w397:dbl)
            n192 = local read "I 2probe [nA]"() -> (w372:dbl)
            n193 = local read "DAC 1 V [V]"() -> (w353:dbl)
            n194 = local read "DAC 2 V [V]"() -> (w351:dbl)
            n195 = local read "DAC 3 V [V]"() -> (w345:dbl)
            n196 = local read "DAC 4 V [V]"() -> (w344:dbl)
            n197 = local read "K2400 1 [V]"() -> (w403:dbl)
            n198 = local read "K2400 2 [V]"() -> (w401:dbl)
            n199 = local read "T [K]"() -> (w407:dbl)
            n200 = local read "Time [s]"() -> (w409:dbl)
            n201 = local read "Vsd [V]"() -> (w380:dbl)
            n202 = local read "Vxy [V]"() -> (w363:dbl)
            n203 = local read "Vxx [V]"() -> (w364:dbl)
            n204 = Array Size(array=w338) -> (size(s)=w339:i32)
            n205 = local read "B [T]"() -> (w405:dbl)
            n206 = for {
              N: w339 -> [_]
              tunnel: w338 -> [w414] mode=indexing
              tunnel: [w412] -> w337 mode=indexing
              n207 = Number To Exponential String(number=w414) -> (E-format string=w413:string)  [unwired: 3 in]
              n208 = Concatenate Strings(w413, "\t") -> (w412:string)
            }
            n209 = Number To Exponential String(number=w409) -> (E-format string=w408:string)  [unwired: 3 in]
            n210 = Number To Exponential String(number=w407) -> (E-format string=w406:string)  [unwired: 3 in]
            n211 = Number To Exponential String(number=w405) -> (E-format string=w404:string)  [unwired: 3 in]
            n212 = Number To Exponential String(number=w383) -> (E-format string=w382:string)  [unwired: 3 in]
            n213 = Number To Exponential String(number=w380) -> (E-format string=w379:string)  [unwired: 3 in]
            n214 = Number To Exponential String(number=w378) -> (E-format string=w376:string)  [unwired: 3 in]
            n215 = Number To Exponential String(number=w377) -> (E-format string=w375:string)  [unwired: 3 in]
            n216 = Number To Exponential String(number=w372) -> (E-format string=w366:string)  [unwired: 3 in]
            n217 = Number To Exponential String(number=w370) -> (E-format string=w368:string)  [unwired: 3 in]
            n218 = Number To Exponential String(number=w371) -> (E-format string=w369:string)  [unwired: 3 in]
            n219 = Number To Exponential String(number=w364) -> (E-format string=w360:string)  [unwired: 3 in]
            n220 = Number To Exponential String(number=w363) -> (E-format string=w359:string)  [unwired: 3 in]
            n221 = Number To Exponential String(number=w362) -> (E-format string=w358:string)  [unwired: 3 in]
            n222 = Number To Exponential String(number=w361) -> (E-format string=w357:string)  [unwired: 3 in]
            n223 = Number To Exponential String(number=w353) -> (E-format string=w352:string)  [unwired: 3 in]
            n224 = Number To Exponential String(number=w351) -> (E-format string=w350:string)  [unwired: 3 in]
            n225 = Number To Exponential String(number=w345) -> (E-format string=w343:string)  [unwired: 3 in]
            n226 = Number To Exponential String(number=w344) -> (E-format string=w342:string)  [unwired: 3 in]
            n227 = Number To Exponential String(number=w403) -> (E-format string=w402:string)  [unwired: 3 in]
            n228 = Number To Exponential String(number=w401) -> (E-format string=w400:string)  [unwired: 3 in]
            n229 = Number To Exponential String(number=w399) -> (E-format string=w398:string)  [unwired: 3 in]
            n230 = Concatenate Strings(w379, w374, w376, w374, w375, w374) -> (w373:string)
            n231 = Concatenate Strings(w352, w341, w350, w341, w343, w341, w342, w341, w402, w341, w400, w341, w398, w341) -> (w340:string)
            n232 = Concatenate Strings(w366, w367, w368, w367, w369, w367) -> (w365:string)
            n233 = Concatenate Strings(w360, w356, w359, w356, w358, w356, w357) -> (w355:string)
            n234 = Concatenate Strings(w408, w381, w406, w381, w404, w381, w382, w381) -> (w346:string)
            n235 = local read "refnum data"() -> (w410:refnum<file>)
            n236 = Concatenate Strings(w346, w373, w365, w355, w334) -> (w384:string)
            n237 = Write to Text File(file (use dialog)=w410, text=w384) -> (error out=w348:errorcluster)  [unwired: 1 in, 3 out]
            n238 = local read "Lockin1 Y [V]"() -> (w396:dbl)
            n239 = local read "Lockin2 X [V]"() -> (w395:dbl)
            n240 = local read "Lockin2 Y [V]"() -> (w394:dbl)
            n241 = local read "I K2400_1 [A]"() -> (w388:dbl)
            n242 = local read "I K2400_2 [A]"() -> (w387:dbl)
            n243 = Number To Exponential String(number=w397) -> (E-format string=w393:string)  [unwired: 3 in]
            n244 = Number To Exponential String(number=w396) -> (E-format string=w392:string)  [unwired: 3 in]
            n245 = Number To Exponential String(number=w395) -> (E-format string=w391:string)  [unwired: 3 in]
            n246 = Number To Exponential String(number=w394) -> (E-format string=w390:string)  [unwired: 3 in]
            n247 = Number To Exponential String(number=w388) -> (E-format string=w386:string)  [unwired: 3 in]
            n248 = Number To Exponential String(number=w387) -> (E-format string=w385:string)  [unwired: 3 in]
            n249 = Concatenate Strings(w393, w389, w392, w389, w391, w389, w390, w389) -> (w335:string)
            n250 = Concatenate Strings(w337, w386, w354, w385, w354) -> (w336:string)
            n251 = local read "refnum raw"() -> (w349:refnum<file>)
            n252 = Concatenate Strings(w346, w340, w335, w336, w334) -> (w347:string)
            n253 = Write to Text File(file (use dialog)=w349, text=w347, error in=w348) -> ()  [unwired: 4 out]
          }
        }
        n254 = local read "Refresh Rate [ms]"() -> (w332:i32)
        n255 = call "wait.vi"("wait time (ms)"=w332) -> ("error in (no error) 2"=w331:errorcluster)  [unwired: 1 in]
      }
      frame "Calculate" {
        w439 = string[] ["Temperature", "B", "Wavelength", "Vsd", "Isd", "Vbg", "Vtg", "Ibg", "Itg", "Vxx", "Vxy", "R2probe", "R4probe", "Rxy"] ("Axis select")
        # "lockin1 X\nLockin2 X\nI K2400 01\nI K2400 02\nDMMxxx"
        # "DAC 1\nK2400 1\nK2400 2\nLockin\nDAC 2\nDAC 3\nDAC 4"
        n256 = local read "Gain Cluster 2"() -> (w478:T3)
        n257 = local read "SetIntr Cluster"() -> (w416:cluster{dbl, dbl, dbl, dbl, dbl, dbl, dbl})
        n258 = local read "signal cluster"() -> (w417:T5)
        n259 = Unbundle By Name(w478) -> ("Vsd"=w420:string, "I 2probe 2"=w418:string, "Vxx"=w423:string, "Vxy"=w421:string, "V BG"=w432:string, "I leak BG"=w428:string, "V TG"=w430:string, "I leak TG"=w426:string)
        n260 = Unbundle By Name(w478) -> ("I Gain 1"=w490:dbl, "V Gain 1"=w494:dbl, "conversion factor BG"=w492:dbl, "Vin / Vout 1"=w493:dbl, "V Gain 2"=w484:dbl, "Vin / Vout 2"=w483:dbl, "V Gain 3"=w482:dbl, "Vin / Vout 3"=w481:dbl, "I Gain 2"=w486:dbl, "I Gain 3"=w489:dbl, "conversion factor TG"=w480:dbl, "Vin / Vout 4"=w491:dbl, "Vin / Vout 5"=w479:dbl, "Manual Gain 1"=w485:dbl, "Manual Gain 2"=w487:dbl, "Manual Gain 3"=w488:dbl)
        n261 = call "SignalOutput.vi"("signal cluster"=w417, "Gain Type"=w432, "SetIntr Cluster"=w416) -> ("Signal output"=w431:dbl)
        n262 = call "SignalOutput.vi"("signal cluster"=w417, "Gain Type"=w430, "SetIntr Cluster"=w416) -> ("Signal output"=w429:dbl)
        n263 = call "SignalOutput.vi"("signal cluster"=w417, "Gain Type"=w428, "SetIntr Cluster"=w416) -> ("Signal output"=w427:dbl)
        n264 = call "SignalOutput.vi"("signal cluster"=w417, "Gain Type"=w426, "SetIntr Cluster"=w416) -> ("Signal output"=w425:dbl)
        n265 = call "SignalOutput.vi"("signal cluster"=w417, "Gain Type"=w423, "SetIntr Cluster"=w416) -> ("Signal output"=w424:dbl)
        n266 = call "SignalOutput.vi"("signal cluster"=w417, "Gain Type"=w420, "SetIntr Cluster"=w416) -> ("Signal output"=w419:dbl)
        n267 = call "SignalOutput.vi"("signal cluster"=w417, "Gain Type"=w421, "SetIntr Cluster"=w416) -> ("Signal output"=w422:dbl)
        n268 = call "SignalOutput.vi"("signal cluster"=w417, "Gain Type"=w418, "SetIntr Cluster"=w416) -> ("Signal output"=w415:dbl)
        n269 = Multiply(x=w431, y=w492) -> (x*y=w513:dbl)
        n270 = Multiply(x=w429, y=w480) -> (x*y=w512:dbl)
        n271 = Divide(x=w427, y=w486) -> (x/y=w517:dbl)
        n272 = Divide(x=w425, y=w489) -> (x/y=w516:dbl)
        n273 = Divide(x=w424, y=w484) -> (x/y=w515:dbl)
        n274 = Multiply(x=w494, y=w419) -> (x*y=w520:dbl)
        n275 = Divide(x=w422, y=w482) -> (x/y=w514:dbl)
        n276 = Divide(x=w415, y=w490) -> (x/y=w518:dbl)
        n277 = Multiply(x=w517, y=w487) -> (x*y=w497:dbl)
        n278 = Multiply(x=w516, y=w488) -> (x*y=w509:dbl)
        n279 = Multiply(x=w513, y=w491) -> (x*y=w503:dbl)
        "V_backgate [V]" <- w503
        n280 = Multiply(x=w512, y=w479) -> (x*y=w501:dbl)
        "V_topgate [V]" <- w501
        n281 = Multiply(x=w515, y=w483) -> (x*y=w505:dbl)
        "Vxx [V]" <- w505
        n282 = Multiply(x=w520, y=w493) -> (x*y=w511:dbl)
        "Vsd [V]" <- w511
        n283 = Multiply(x=w514, y=w481) -> (x*y=w470:dbl)
        "Vxy [V]" <- w470
        n284 = Multiply(x=w518, y=w485) -> (x*y=w468:dbl)
        n285 = Multiply(x=w497, y=1000000000.0) -> (x*y=w496:dbl)
        "I Leak BG [nA]" <- w496
        n286 = Multiply(x=w509, y=1000000000.0) -> (x*y=w500:dbl)
        "I Leak TG[nA]" <- w500
        n287 = Multiply(x=w468, y=1000000000.0) -> (x*y=w469:dbl)
        "I 2probe [nA]" <- w469
        n288 = Divide(x=w511, y=w469) -> (x/y=w477:dbl)
        n289 = Divide(x=w505, y=w469) -> (x/y=w473:dbl)
        n290 = Divide(x=w470, y=w468) -> (x/y=w467:dbl)
        n291 = Divide(x=w467, y=1000.0) -> (x/y=w465:dbl)
        n292 = local read "R2probe array"() -> (w507:dbl[])
        n293 = local read "R4probe array"() -> (w506:dbl[])
        n294 = local read "Vbg array"() -> (w459:dbl[])
        n295 = local read "Vsd array"() -> (w461:dbl[])
        n296 = local read "Rxy Array"() -> (w471:dbl[])
        n297 = local read "Vtg array"() -> (w458:dbl[])
        n298 = local read "Ibg array"() -> (w508:dbl[])
        n299 = local read "Vxx array"() -> (w504:dbl[])
        n300 = local read "Vxy array"() -> (w502:dbl[])
        n301 = local read "Isd array"() -> (w460:dbl[])
        n302 = local read "Itg array"() -> (w510:dbl[])
        n303 = Multiply(x=w477, y=1000000.0) -> (x*y=w475:dbl)
        "R 2probe [kOhm]" <- w475
        n304 = Multiply(x=w473, y=1000000.0) -> (x*y=w472:dbl)
        "R 4probe [kOhm]" <- w472
        n305 = local read "Wavelength array"() -> (w462:dbl[])
        n306 = Build Array (concatenate)(w461, w511) -> (w457:dbl[])
        n307 = Build Array (concatenate)(w460, w469) -> (w456:dbl[])
        n308 = Build Array (concatenate)(w459, w503) -> (w455:dbl[])
        n309 = Build Array (concatenate)(w458, w501) -> (w454:dbl[])
        n310 = Build Array (concatenate)(w508, w496) -> (w453:dbl[])
        n311 = Build Array (concatenate)(w510, w500) -> (w452:dbl[])
        n312 = Build Array (concatenate)(w504, w505) -> (w451:dbl[])
        n313 = Build Array (concatenate)(w502, w470) -> (w450:dbl[])
        n314 = Build Array (concatenate)(w507, w475) -> (w449:dbl[])
        n315 = Build Array (concatenate)(w506, w472) -> (w448:dbl[])
        n316 = Build Array (concatenate)(w471, w465) -> (w447:dbl[])
        n317 = local write "R4probe array"(w448) -> ()
        n318 = local write "Ibg array"(w453) -> ()
        n319 = local write "Itg array"(w452) -> ()
        n320 = local read "T"() -> (w464:dbl[])
        n321 = local read "B"() -> (w463:dbl[])
        n322 = local write "Vsd array"(w457) -> ()
        n323 = local write "Vxy array"(w450) -> ()
        n324 = local write "R2probe array"(w449) -> ()
        n325 = local write "Rxy Array"(w447) -> ()
        n326 = local write "Vbg array"(w455) -> ()
        n327 = local write "Vtg array"(w454) -> ()
        n328 = local write "Vxx array"(w451) -> ()
        n329 = local write "Isd array"(w456) -> ()
        n330 = Build Array(w464, w463, w462, w457, w456, w455, w454, w453, w452, w451, w450, w449, w448, w447) -> (w440:dbl[][])
        n331 = call "Evalmutlivar.vi"("Variables"=w439, "Matrix data"=w440, "formula"="Formula 2") -> ("error out"=w435:errorcluster, "Y Values"=→"Formula2Array":dbl[])  [unwired: 1 in]
        n332 = call "Evalmutlivar.vi"("Variables"=w439, "Matrix data"=w440, "formula"="Formula 3") -> ("error out"=w434:errorcluster, "Y Values"=→"Formula3Array":dbl[])  [unwired: 1 in]
        n333 = call "Evalmutlivar.vi"("Variables"=w439, "Matrix data"=w440, "formula"="Formula 4") -> ("error out"=w433:errorcluster, "Y Values"=→"Formula4Array":dbl[])  [unwired: 1 in]
        n334 = call "Evalmutlivar.vi"("Variables"=w439, "Matrix data"=w440, "formula"="Formula 1") -> ("error out"=w445:errorcluster, "Y Values"=→"Formula1Array":dbl[])  [unwired: 1 in]
      }
      frame "stop" {
        n335 = local read "refnum data"() -> (w521:refnum<file>)
        n336 = Close File(refnum=w521) -> ()  [unwired: 1 in, 2 out]
      }
    }
    n337 = global read "stopButton.vi" "stopsignal"() -> (w31:bool)
    n338 = local write "stop"(w31) -> ()
    n339 = Unbundle By Name("Device Cluster") -> ("K2400 1"=→"K2400 1":refnum<visa-resource-name>, "K2400_1"=→"K2400_1":bool, "K2400 2"=→"K2400 2":refnum<visa-resource-name>, "K2400_2"=→"K2400_2":bool, "Lockin1"=→"Lockin1":refnum<visa-resource-name>, "Lockin1 present"=→"Lockin1 present":bool, "Lockin2"=→"Lockin2":refnum<visa-resource-name>, "Lockin2 present"=→"Lockin2 present":bool, "TIC"=→"TIC":refnum<visa-resource-name>, "Tcontrol"=→"Tcontrol":string, "DMMX"=→"DMMX":string[][], "DAC"=→"DAC":refnum<visa-resource-name>, "DAC present"=→"DAC present":bool, "Bfield query"=→"Bfield query":bool, "Wvlen query"=→"Wvlen query":bool, "ITC signal"=→"ITC signal":T1)
    n340 = Or(x=w34, y="stop") -> (x .or. y?=w32:bool)
    "stopMainLoop" <- w32
  }
  n341 = Array Size(array=w7) -> (size(s)=w8:i32[])
  n342 = Index Array(array=w8, index=0) -> (element=w6:i32)
  n343 = for {
    N: w6 -> [_]
    tunnel: w7 -> [_] mode=indexing
    tunnel: [w524] -> w4 mode=indexing
    i -> [w527]
    n344 = Increment(x=w527) -> (x+1=w525:i32)
    n345 = Number To Decimal String(number=w525) -> (decimal integer string=w526:string)  [unwired: 1 in]
    n346 = Concatenate Strings("DMM", w526) -> (w524:string)
  }
  n347 = while {
    shift-right: [w569] -> _
    shift-left: "plot" -> [w570]
    tunnel: w2 -> [w530]
    tunnel: w1 -> [w529]
    stop <- w571 stop-if-true
    n348 = local read "Refresh Rate [ms]"() -> (w533:i32)
    n349 = local read "stopMainLoop"() -> (w571:bool)
    n350 = case shown="\"DMM1\"..\"DMM9\"" "Y-Axis 2" {
      selector: "Y-Axis 2" -> [_ _ _ _ _ _ _ _ _ _ _ _ _ _ _ _ _ _ _ _ _ _ _ w677 _ _ _ _ _ _]
      tunnel: [w647 w648 w649 w650 w651 w652 w653 w654 w655 w656 w657 w658 w659 w660 w661 w662 w663 w664 w665 w666 w667 w668 w669 w671 w678 w679 w680 w681 w682 w683] -> w539
      frame "DAC 1 V", Default {
        n351 = local read "DAC 1 array"() -> (w647:dbl[])
      }
      frame "DAC 2 V" {
        n352 = local read "DAC 2 array"() -> (w648:dbl[])
      }
      frame "Wavelength" {
        n353 = local read "Wavelength array"() -> (w649:dbl[])
      }
      frame "Vsd" {
        n354 = local read "Vsd array"() -> (w650:dbl[])
      }
      frame "Isd" {
        n355 = local read "Isd array"() -> (w651:dbl[])
      }
      frame "Vbg" {
        n356 = local read "Vbg array"() -> (w652:dbl[])
      }
      frame "Vtg" {
        n357 = local read "Vtg array"() -> (w653:dbl[])
      }
      frame "Ibg" {
        n358 = local read "Ibg array"() -> (w654:dbl[])
      }
      frame "Itg" {
        n359 = local read "Ibg array"() -> (w655:dbl[])
      }
      frame "Vxx" {
        n360 = local read "Vxx array"() -> (w656:dbl[])
      }
      frame "Vxy" {
        n361 = local read "Vxy array"() -> (w657:dbl[])
      }
      frame "Rxy" {
        n362 = local read "Rxy Array"() -> (w658:dbl[])
      }
      frame "R2probe" {
        n363 = local read "R2probe array"() -> (w659:dbl[])
      }
      frame "Temperature" {
        n364 = local read "T"() -> (w660:dbl[])
      }
      frame "time" {
        n365 = local read "Time"() -> (w661:dbl[])
      }
      frame "Lockin1 X" {
        n366 = local read "Lockin1 X"() -> (w662:dbl[])
      }
      frame "Lockin2 X" {
        n367 = local read "Lockin2 X"() -> (w663:dbl[])
      }
      frame "Lockin1 Y" {
        n368 = local read "Lockin1 Y"() -> (w664:dbl[])
      }
      frame "Lockin2 Y" {
        n369 = local read "Lockin2 Y"() -> (w665:dbl[])
      }
      frame "V K2400_01" {
        n370 = local read "V K2400_01 array"() -> (w666:dbl[])
      }
      frame "V K2400_02" {
        n371 = local read "V K2400_02 array"() -> (w667:dbl[])
      }
      frame "I K2400_01" {
        n372 = local read "I K2400 01"() -> (w668:dbl[])
      }
      frame "I K2400_02" {
        n373 = local read "I K2400 02"() -> (w669:dbl[])
      }
      frame "DMM1".."DMM9" {
        n374 = Match Pattern(string=w677, regular expression="DMM") -> (after substring=w675:string)  [unwired: 1 in, 3 out]
        n375 = Scan Value(string=w675, format string="%g") -> (value=w672:dbl)  [unwired: 1 in, 1 out]
        n376 = local read "DMM Array"() -> (w673:dbl[][])
        n377 = Decrement(x=w672) -> (x-1=w670:dbl)
        n378 = Index Array(array=w673, index (col)=w670) -> (element=w671:dbl[])  [unwired: 1 in]
      }
      frame "B" {
        n379 = local read "B"() -> (w678:dbl[])
      }
      frame "R4probe" {
        n380 = local read "R4probe array"() -> (w679:dbl[])
      }
      frame "Formula1" {
        n381 = local read "Formula1Array"() -> (w680:dbl[])
      }
      frame "Formula2" {
        n382 = local read "Formula2Array"() -> (w681:dbl[])
      }
      frame "Formula3" {
        n383 = local read "Formula3Array"() -> (w682:dbl[])
      }
      frame "Formula4" {
        n384 = local read "Formula4Array"() -> (w683:dbl[])
      }
    }
    n385 = call "AxisLabel.vi"("Axis"="X-Axis 2") -> ("X Scale.Name Label.Text"=w567:string)
    n386 = case shown="\"DMM1\"..\"DMM9\"" "X-Axis 2" {
      selector: "X-Axis 2" -> [_ _ _ _ _ _ _ _ _ _ _ _ _ _ _ _ _ _ _ _ _ _ _ w714 _ _ _ _ _ _]
      tunnel: [w684 w685 w686 w687 w688 w689 w690 w691 w692 w693 w694 w695 w696 w697 w698 w699 w700 w701 w702 w703 w704 w705 w706 w708 w715 w716 w717 w718 w719 w720] -> w540
      frame "DAC 1 V", Default {
        n387 = local read "DAC 1 array"() -> (w684:dbl[])
      }
      frame "DAC 2 V" {
        n388 = local read "DAC 2 array"() -> (w685:dbl[])
      }
      frame "Wavelength" {
        n389 = local read "Wavelength array"() -> (w686:dbl[])
      }
      frame "Vsd" {
        n390 = local read "Vsd array"() -> (w687:dbl[])
      }
      frame "Isd" {
        n391 = local read "Isd array"() -> (w688:dbl[])
      }
      frame "Vbg" {
        n392 = local read "Vbg array"() -> (w689:dbl[])
      }
      frame "Vtg" {
        n393 = local read "Vtg array"() -> (w690:dbl[])
      }
      frame "Ibg" {
        n394 = local read "Ibg array"() -> (w691:dbl[])
      }
      frame "Itg" {
        n395 = local read "Ibg array"() -> (w692:dbl[])
      }
      frame "Vxx" {
        n396 = local read "Vxx array"() -> (w693:dbl[])
      }
      frame "Vxy" {
        n397 = local read "Vxy array"() -> (w694:dbl[])
      }
      frame "Rxy" {
        n398 = local read "Rxy Array"() -> (w695:dbl[])
      }
      frame "R2probe" {
        n399 = local read "R2probe array"() -> (w696:dbl[])
      }
      frame "Temperature" {
        n400 = local read "T"() -> (w697:dbl[])
      }
      frame "time" {
        n401 = local read "Time"() -> (w698:dbl[])
      }
      frame "Lockin1 X" {
        n402 = local read "Lockin1 X"() -> (w699:dbl[])
      }
      frame "Lockin2 X" {
        n403 = local read "Lockin2 X"() -> (w700:dbl[])
      }
      frame "Lockin1 Y" {
        n404 = local read "Lockin1 Y"() -> (w701:dbl[])
      }
      frame "Lockin2 Y" {
        n405 = local read "Lockin2 Y"() -> (w702:dbl[])
      }
      frame "V K2400_01" {
        n406 = local read "V K2400_01 array"() -> (w703:dbl[])
      }
      frame "V K2400_02" {
        n407 = local read "V K2400_02 array"() -> (w704:dbl[])
      }
      frame "I K2400_01" {
        n408 = local read "I K2400 01"() -> (w705:dbl[])
      }
      frame "I K2400_02" {
        n409 = local read "I K2400 02"() -> (w706:dbl[])
      }
      frame "DMM1".."DMM9" {
        n410 = Match Pattern(string=w714, regular expression="DMM") -> (after substring=w712:string)  [unwired: 1 in, 3 out]
        n411 = Scan Value(string=w712, format string="%g") -> (value=w709:dbl)  [unwired: 1 in, 1 out]
        n412 = local read "DMM Array"() -> (w710:dbl[][])
        n413 = Decrement(x=w709) -> (x-1=w707:dbl)
        n414 = Index Array(array=w710, index (col)=w707) -> (element=w708:dbl[])  [unwired: 1 in]
      }
      frame "B" {
        n415 = local read "B"() -> (w715:dbl[])
      }
      frame "R4probe" {
        n416 = local read "R4probe array"() -> (w716:dbl[])
      }
      frame "Formula1" {
        n417 = local read "Formula1Array"() -> (w717:dbl[])
      }
      frame "Formula2" {
        n418 = local read "Formula2Array"() -> (w718:dbl[])
      }
      frame "Formula3" {
        n419 = local read "Formula3Array"() -> (w719:dbl[])
      }
      frame "Formula4" {
        n420 = local read "Formula4Array"() -> (w720:dbl[])
      }
    }
    n421 = case shown="\"DMM1\"..\"DMM9\"" "X-Axis 1" {
      selector: "X-Axis 1" -> [_ _ _ _ _ _ _ _ _ _ _ _ _ _ _ _ _ _ _ _ _ _ _ w640 _ _ _ _ _ _]
      tunnel: [w610 w611 w612 w613 w614 w615 w616 w617 w618 w619 w620 w621 w622 w623 w624 w625 w626 w627 w628 w629 w630 w631 w632 w634 w641 w642 w643 w644 w645 w646] -> w537
      frame "DAC 1 V", Default {
        n422 = local read "DAC 1 array"() -> (w610:dbl[])
      }
      frame "DAC 2 V" {
        n423 = local read "DAC 2 array"() -> (w611:dbl[])
      }
      frame "Wavelength" {
        n424 = local read "Wavelength array"() -> (w612:dbl[])
      }
      frame "Vsd" {
        n425 = local read "Vsd array"() -> (w613:dbl[])
      }
      frame "Isd" {
        n426 = local read "Isd array"() -> (w614:dbl[])
      }
      frame "Vbg" {
        n427 = local read "Vbg array"() -> (w615:dbl[])
      }
      frame "Vtg" {
        n428 = local read "Vtg array"() -> (w616:dbl[])
      }
      frame "Ibg" {
        n429 = local read "Ibg array"() -> (w617:dbl[])
      }
      frame "Itg" {
        n430 = local read "Ibg array"() -> (w618:dbl[])
      }
      frame "Vxx" {
        n431 = local read "Vxx array"() -> (w619:dbl[])
      }
      frame "Vxy" {
        n432 = local read "Vxy array"() -> (w620:dbl[])
      }
      frame "Rxy" {
        n433 = local read "Rxy Array"() -> (w621:dbl[])
      }
      frame "R2probe" {
        n434 = local read "R2probe array"() -> (w622:dbl[])
      }
      frame "Temperature" {
        n435 = local read "T"() -> (w623:dbl[])
      }
      frame "time" {
        n436 = local read "Time"() -> (w624:dbl[])
      }
      frame "Lockin1 X" {
        n437 = local read "Lockin1 X"() -> (w625:dbl[])
      }
      frame "Lockin2 X" {
        n438 = local read "Lockin2 X"() -> (w626:dbl[])
      }
      frame "Lockin1 Y" {
        n439 = local read "Lockin1 Y"() -> (w627:dbl[])
      }
      frame "Lockin2 Y" {
        n440 = local read "Lockin2 Y"() -> (w628:dbl[])
      }
      frame "V K2400_01" {
        n441 = local read "V K2400_01 array"() -> (w629:dbl[])
      }
      frame "V K2400_02" {
        n442 = local read "V K2400_02 array"() -> (w630:dbl[])
      }
      frame "I K2400_01" {
        n443 = local read "I K2400 01"() -> (w631:dbl[])
      }
      frame "I K2400_02" {
        n444 = local read "I K2400 02"() -> (w632:dbl[])
      }
      frame "DMM1".."DMM9" {
        n445 = Match Pattern(string=w640, regular expression="DMM") -> (after substring=w638:string)  [unwired: 1 in, 3 out]
        n446 = Scan Value(string=w638, format string="%g") -> (value=w635:dbl)  [unwired: 1 in, 1 out]
        n447 = local read "DMM Array"() -> (w636:dbl[][])
        n448 = Decrement(x=w635) -> (x-1=w633:dbl)
        n449 = Index Array(array=w636, index (col)=w633) -> (element=w634:dbl[])  [unwired: 1 in]
      }
      frame "B" {
        n450 = local read "B"() -> (w641:dbl[])
      }
      frame "R4probe" {
        n451 = local read "R4probe array"() -> (w642:dbl[])
      }
      frame "Formula1" {
        n452 = local read "Formula1Array"() -> (w643:dbl[])
      }
      frame "Formula2" {
        n453 = local read "Formula2Array"() -> (w644:dbl[])
      }
      frame "Formula3" {
        n454 = local read "Formula3Array"() -> (w645:dbl[])
      }
      frame "Formula4" {
        n455 = local read "Formula4Array"() -> (w646:dbl[])
      }
    }
    n456 = case shown="\"DMM1\"..\"DMM9\"" "Y-Axis 1" {
      selector: "Y-Axis 1" -> [_ _ _ _ _ _ _ _ _ _ _ _ _ _ _ _ _ _ _ _ _ _ _ w603 _ _ _ _ _ _]
      tunnel: [w573 w574 w575 w576 w577 w578 w579 w580 w581 w582 w583 w584 w585 w586 w587 w588 w589 w590 w591 w592 w593 w594 w595 w597 w604 w605 w606 w607 w608 w609] -> w535
      frame "DAC 1 V", Default {
        n457 = local read "DAC 1 array"() -> (w573:dbl[])
      }
      frame "DAC 2 V" {
        n458 = local read "DAC 2 array"() -> (w574:dbl[])
      }
      frame "Wavelength" {
        n459 = local read "Wavelength array"() -> (w575:dbl[])
      }
      frame "Vsd" {
        n460 = local read "Vsd array"() -> (w576:dbl[])
      }
      frame "Isd" {
        n461 = local read "Isd array"() -> (w577:dbl[])
      }
      frame "Vbg" {
        n462 = local read "Vbg array"() -> (w578:dbl[])
      }
      frame "Vtg" {
        n463 = local read "Vtg array"() -> (w579:dbl[])
      }
      frame "Ibg" {
        n464 = local read "Ibg array"() -> (w580:dbl[])
      }
      frame "Itg" {
        n465 = local read "Ibg array"() -> (w581:dbl[])
      }
      frame "Vxx" {
        n466 = local read "Vxx array"() -> (w582:dbl[])
      }
      frame "Vxy" {
        n467 = local read "Vxy array"() -> (w583:dbl[])
      }
      frame "Rxy" {
        n468 = local read "Rxy Array"() -> (w584:dbl[])
      }
      frame "R2probe" {
        n469 = local read "R2probe array"() -> (w585:dbl[])
      }
      frame "Temperature" {
        n470 = local read "T"() -> (w586:dbl[])
      }
      frame "time" {
        n471 = local read "Time"() -> (w587:dbl[])
      }
      frame "Lockin1 X" {
        n472 = local read "Lockin1 X"() -> (w588:dbl[])
      }
      frame "Lockin2 X" {
        n473 = local read "Lockin2 X"() -> (w589:dbl[])
      }
      frame "Lockin1 Y" {
        n474 = local read "Lockin1 Y"() -> (w590:dbl[])
      }
      frame "Lockin2 Y" {
        n475 = local read "Lockin2 Y"() -> (w591:dbl[])
      }
      frame "V K2400_01" {
        n476 = local read "V K2400_01 array"() -> (w592:dbl[])
      }
      frame "V K2400_02" {
        n477 = local read "V K2400_02 array"() -> (w593:dbl[])
      }
      frame "I K2400_01" {
        n478 = local read "I K2400 01"() -> (w594:dbl[])
      }
      frame "I K2400_02" {
        n479 = local read "I K2400 02"() -> (w595:dbl[])
      }
      frame "DMM1".."DMM9" {
        n480 = Match Pattern(string=w603, regular expression="DMM") -> (after substring=w601:string)  [unwired: 1 in, 3 out]
        n481 = Scan Value(string=w601, format string="%g") -> (value=w598:dbl)  [unwired: 1 in, 1 out]
        n482 = local read "DMM Array"() -> (w599:dbl[][])
        n483 = Decrement(x=w598) -> (x-1=w596:dbl)
        n484 = Index Array(array=w599, index (col)=w596) -> (element=w597:dbl[])  [unwired: 1 in]
      }
      frame "B" {
        n485 = local read "B"() -> (w604:dbl[])
      }
      frame "R4probe" {
        n486 = local read "R4probe array"() -> (w605:dbl[])
      }
      frame "Formula1" {
        n487 = local read "Formula1Array"() -> (w606:dbl[])
      }
      frame "Formula2" {
        n488 = local read "Formula2Array"() -> (w607:dbl[])
      }
      frame "Formula3" {
        n489 = local read "Formula3Array"() -> (w608:dbl[])
      }
      frame "Formula4" {
        n490 = local read "Formula4Array"() -> (w609:dbl[])
      }
    }
    n491 = case shown="\"DMM1\"..\"DMM9\"" "X-Axis 3" {
      selector: "X-Axis 3" -> [_ _ _ _ _ _ _ _ _ _ _ _ _ _ _ _ _ _ _ _ _ _ _ w751 _ _ _ _ _ _]
      tunnel: [w721 w722 w723 w724 w725 w726 w727 w728 w729 w730 w731 w732 w733 w734 w735 w736 w737 w738 w739 w740 w741 w742 w743 w745 w752 w753 w754 w755 w756 w757] -> w543
      frame "DAC 1 V", Default {
        n492 = local read "DAC 1 array"() -> (w721:dbl[])
      }
      frame "DAC 2 V" {
        n493 = local read "DAC 2 array"() -> (w722:dbl[])
      }
      frame "Wavelength" {
        n494 = local read "Wavelength array"() -> (w723:dbl[])
      }
      frame "Vsd" {
        n495 = local read "Vsd array"() -> (w724:dbl[])
      }
      frame "Isd" {
        n496 = local read "Isd array"() -> (w725:dbl[])
      }
      frame "Vbg" {
        n497 = local read "Vbg array"() -> (w726:dbl[])
      }
      frame "Vtg" {
        n498 = local read "Vtg array"() -> (w727:dbl[])
      }
      frame "Ibg" {
        n499 = local read "Ibg array"() -> (w728:dbl[])
      }
      frame "Itg" {
        n500 = local read "Ibg array"() -> (w729:dbl[])
      }
      frame "Vxx" {
        n501 = local read "Vxx array"() -> (w730:dbl[])
      }
      frame "Vxy" {
        n502 = local read "Vxy array"() -> (w731:dbl[])
      }
      frame "Rxy" {
        n503 = local read "Rxy Array"() -> (w732:dbl[])
      }
      frame "R2probe" {
        n504 = local read "R2probe array"() -> (w733:dbl[])
      }
      frame "Temperature" {
        n505 = local read "T"() -> (w734:dbl[])
      }
      frame "time" {
        n506 = local read "Time"() -> (w735:dbl[])
      }
      frame "Lockin1 X" {
        n507 = local read "Lockin1 X"() -> (w736:dbl[])
      }
      frame "Lockin2 X" {
        n508 = local read "Lockin2 X"() -> (w737:dbl[])
      }
      frame "Lockin1 Y" {
        n509 = local read "Lockin1 Y"() -> (w738:dbl[])
      }
      frame "Lockin2 Y" {
        n510 = local read "Lockin2 Y"() -> (w739:dbl[])
      }
      frame "V K2400_01" {
        n511 = local read "V K2400_01 array"() -> (w740:dbl[])
      }
      frame "V K2400_02" {
        n512 = local read "V K2400_02 array"() -> (w741:dbl[])
      }
      frame "I K2400_01" {
        n513 = local read "I K2400 01"() -> (w742:dbl[])
      }
      frame "I K2400_02" {
        n514 = local read "I K2400 02"() -> (w743:dbl[])
      }
      frame "DMM1".."DMM9" {
        n515 = Match Pattern(string=w751, regular expression="DMM") -> (after substring=w749:string)  [unwired: 1 in, 3 out]
        n516 = Scan Value(string=w749, format string="%g") -> (value=w746:dbl)  [unwired: 1 in, 1 out]
        n517 = local read "DMM Array"() -> (w747:dbl[][])
        n518 = Decrement(x=w746) -> (x-1=w744:dbl)
        n519 = Index Array(array=w747, index (col)=w744) -> (element=w745:dbl[])  [unwired: 1 in]
      }
      frame "B" {
        n520 = local read "B"() -> (w752:dbl[])
      }
      frame "R4probe" {
        n521 = local read "R4probe array"() -> (w753:dbl[])
      }
      frame "Formula1" {
        n522 = local read "Formula1Array"() -> (w754:dbl[])
      }
      frame "Formula2" {
        n523 = local read "Formula2Array"() -> (w755:dbl[])
      }
      frame "Formula3" {
        n524 = local read "Formula3Array"() -> (w756:dbl[])
      }
      frame "Formula4" {
        n525 = local read "Formula4Array"() -> (w757:dbl[])
      }
    }
    n526 = case shown="\"DMM1\"..\"DMM9\"" "Y-Axis 3" {
      selector: "Y-Axis 3" -> [_ _ _ _ _ _ _ _ _ _ _ _ _ _ _ _ _ _ _ _ _ _ _ w788 _ _ _ _ _ _]
      tunnel: [w758 w759 w760 w761 w762 w763 w764 w765 w766 w767 w768 w769 w770 w771 w772 w773 w774 w775 w776 w777 w778 w779 w780 w782 w789 w790 w791 w792 w793 w794] -> w545
      frame "DAC 1 V", Default {
        n527 = local read "DAC 1 array"() -> (w758:dbl[])
      }
      frame "DAC 2 V" {
        n528 = local read "DAC 2 array"() -> (w759:dbl[])
      }
      frame "Wavelength" {
        n529 = local read "Wavelength array"() -> (w760:dbl[])
      }
      frame "Vsd" {
        n530 = local read "Vsd array"() -> (w761:dbl[])
      }
      frame "Isd" {
        n531 = local read "Isd array"() -> (w762:dbl[])
      }
      frame "Vbg" {
        n532 = local read "Vbg array"() -> (w763:dbl[])
      }
      frame "Vtg" {
        n533 = local read "Vtg array"() -> (w764:dbl[])
      }
      frame "Ibg" {
        n534 = local read "Ibg array"() -> (w765:dbl[])
      }
      frame "Itg" {
        n535 = local read "Ibg array"() -> (w766:dbl[])
      }
      frame "Vxx" {
        n536 = local read "Vxx array"() -> (w767:dbl[])
      }
      frame "Vxy" {
        n537 = local read "Vxy array"() -> (w768:dbl[])
      }
      frame "Rxy" {
        n538 = local read "Rxy Array"() -> (w769:dbl[])
      }
      frame "R2probe" {
        n539 = local read "R2probe array"() -> (w770:dbl[])
      }
      frame "Temperature" {
        n540 = local read "T"() -> (w771:dbl[])
      }
      frame "time" {
        n541 = local read "Time"() -> (w772:dbl[])
      }
      frame "Lockin1 X" {
        n542 = local read "Lockin1 X"() -> (w773:dbl[])
      }
      frame "Lockin2 X" {
        n543 = local read "Lockin2 X"() -> (w774:dbl[])
      }
      frame "Lockin1 Y" {
        n544 = local read "Lockin1 Y"() -> (w775:dbl[])
      }
      frame "Lockin2 Y" {
        n545 = local read "Lockin2 Y"() -> (w776:dbl[])
      }
      frame "V K2400_01" {
        n546 = local read "V K2400_01 array"() -> (w777:dbl[])
      }
      frame "V K2400_02" {
        n547 = local read "V K2400_02 array"() -> (w778:dbl[])
      }
      frame "I K2400_01" {
        n548 = local read "I K2400 01"() -> (w779:dbl[])
      }
      frame "I K2400_02" {
        n549 = local read "I K2400 02"() -> (w780:dbl[])
      }
      frame "DMM1".."DMM9" {
        n550 = Match Pattern(string=w788, regular expression="DMM") -> (after substring=w786:string)  [unwired: 1 in, 3 out]
        n551 = Scan Value(string=w786, format string="%g") -> (value=w783:dbl)  [unwired: 1 in, 1 out]
        n552 = local read "DMM Array"() -> (w784:dbl[][])
        n553 = Decrement(x=w783) -> (x-1=w781:dbl)
        n554 = Index Array(array=w784, index (col)=w781) -> (element=w782:dbl[])  [unwired: 1 in]
      }
      frame "B" {
        n555 = local read "B"() -> (w789:dbl[])
      }
      frame "R4probe" {
        n556 = local read "R4probe array"() -> (w790:dbl[])
      }
      frame "Formula1" {
        n557 = local read "Formula1Array"() -> (w791:dbl[])
      }
      frame "Formula2" {
        n558 = local read "Formula2Array"() -> (w792:dbl[])
      }
      frame "Formula3" {
        n559 = local read "Formula3Array"() -> (w793:dbl[])
      }
      frame "Formula4" {
        n560 = local read "Formula4Array"() -> (w794:dbl[])
      }
    }
    n561 = call "AxisLabel.vi"("Axis"="X-Axis 3") -> ("X Scale.Name Label.Text"=w557:string)
    n562 = call "AxisLabel.vi"("Axis"="Y-Axis 3") -> ("X Scale.Name Label.Text"=w556:string)
    n563 = case shown="\"DMM1\"..\"DMM9\"" "X-Axis 4" {
      selector: "X-Axis 4" -> [_ _ _ _ _ _ _ _ _ _ _ _ _ _ _ _ _ _ _ _ _ _ _ w862 _ _ _ _ _ _]
      tunnel: [w832 w833 w834 w835 w836 w837 w838 w839 w840 w841 w842 w843 w844 w845 w846 w847 w848 w849 w850 w851 w852 w853 w854 w856 w863 w864 w865 w866 w867 w868] -> w549
      frame "DAC 1 V", Default {
        n564 = local read "DAC 1 array"() -> (w832:dbl[])
      }
      frame "DAC 2 V" {
        n565 = local read "DAC 2 array"() -> (w833:dbl[])
      }
      frame "Wavelength" {
        n566 = local read "Wavelength array"() -> (w834:dbl[])
      }
      frame "Vsd" {
        n567 = local read "Vsd array"() -> (w835:dbl[])
      }
      frame "Isd" {
        n568 = local read "Isd array"() -> (w836:dbl[])
      }
      frame "Vbg" {
        n569 = local read "Vbg array"() -> (w837:dbl[])
      }
      frame "Vtg" {
        n570 = local read "Vtg array"() -> (w838:dbl[])
      }
      frame "Ibg" {
        n571 = local read "Ibg array"() -> (w839:dbl[])
      }
      frame "Itg" {
        n572 = local read "Ibg array"() -> (w840:dbl[])
      }
      frame "Vxx" {
        n573 = local read "Vxx array"() -> (w841:dbl[])
      }
      frame "Vxy" {
        n574 = local read "Vxy array"() -> (w842:dbl[])
      }
      frame "Rxy" {
        n575 = local read "Rxy Array"() -> (w843:dbl[])
      }
      frame "R2probe" {
        n576 = local read "R2probe array"() -> (w844:dbl[])
      }
      frame "Temperature" {
        n577 = local read "T"() -> (w845:dbl[])
      }
      frame "time" {
        n578 = local read "Time"() -> (w846:dbl[])
      }
      frame "Lockin1 X" {
        n579 = local read "Lockin1 X"() -> (w847:dbl[])
      }
      frame "Lockin2 X" {
        n580 = local read "Lockin2 X"() -> (w848:dbl[])
      }
      frame "Lockin1 Y" {
        n581 = local read "Lockin1 Y"() -> (w849:dbl[])
      }
      frame "Lockin2 Y" {
        n582 = local read "Lockin2 Y"() -> (w850:dbl[])
      }
      frame "V K2400_01" {
        n583 = local read "V K2400_01 array"() -> (w851:dbl[])
      }
      frame "V K2400_02" {
        n584 = local read "V K2400_02 array"() -> (w852:dbl[])
      }
      frame "I K2400_01" {
        n585 = local read "I K2400 01"() -> (w853:dbl[])
      }
      frame "I K2400_02" {
        n586 = local read "I K2400 02"() -> (w854:dbl[])
      }
      frame "DMM1".."DMM9" {
        n587 = Match Pattern(string=w862, regular expression="DMM") -> (after substring=w860:string)  [unwired: 1 in, 3 out]
        n588 = Scan Value(string=w860, format string="%g") -> (value=w857:dbl)  [unwired: 1 in, 1 out]
        n589 = local read "DMM Array"() -> (w858:dbl[][])
        n590 = Decrement(x=w857) -> (x-1=w855:dbl)
        n591 = Index Array(array=w858, index (col)=w855) -> (element=w856:dbl[])  [unwired: 1 in]
      }
      frame "B" {
        n592 = local read "B"() -> (w863:dbl[])
      }
      frame "R4probe" {
        n593 = local read "R4probe array"() -> (w864:dbl[])
      }
      frame "Formula1" {
        n594 = local read "Formula1Array"() -> (w865:dbl[])
      }
      frame "Formula2" {
        n595 = local read "Formula2Array"() -> (w866:dbl[])
      }
      frame "Formula3" {
        n596 = local read "Formula3Array"() -> (w867:dbl[])
      }
      frame "Formula4" {
        n597 = local read "Formula4Array"() -> (w868:dbl[])
      }
    }
    n598 = case shown="\"DMM1\"..\"DMM9\"" "Y-Axis 4" {
      selector: "Y-Axis 4" -> [_ _ _ _ _ _ _ _ _ _ _ _ _ _ _ _ _ _ _ _ _ _ _ w825 _ _ _ _ _ _]
      tunnel: [w795 w796 w797 w798 w799 w800 w801 w802 w803 w804 w805 w806 w807 w808 w809 w810 w811 w812 w813 w814 w815 w816 w817 w819 w826 w827 w828 w829 w830 w831] -> w547
      frame "DAC 1 V", Default {
        n599 = local read "DAC 1 array"() -> (w795:dbl[])
      }
      frame "DAC 2 V" {
        n600 = local read "DAC 2 array"() -> (w796:dbl[])
      }
      frame "Wavelength" {
        n601 = local read "Wavelength array"() -> (w797:dbl[])
      }
      frame "Vsd" {
        n602 = local read "Vsd array"() -> (w798:dbl[])
      }
      frame "Isd" {
        n603 = local read "Isd array"() -> (w799:dbl[])
      }
      frame "Vbg" {
        n604 = local read "Vbg array"() -> (w800:dbl[])
      }
      frame "Vtg" {
        n605 = local read "Vtg array"() -> (w801:dbl[])
      }
      frame "Ibg" {
        n606 = local read "Ibg array"() -> (w802:dbl[])
      }
      frame "Itg" {
        n607 = local read "Ibg array"() -> (w803:dbl[])
      }
      frame "Vxx" {
        n608 = local read "Vxx array"() -> (w804:dbl[])
      }
      frame "Vxy" {
        n609 = local read "Vxy array"() -> (w805:dbl[])
      }
      frame "Rxy" {
        n610 = local read "Rxy Array"() -> (w806:dbl[])
      }
      frame "R2probe" {
        n611 = local read "R2probe array"() -> (w807:dbl[])
      }
      frame "Temperature" {
        n612 = local read "T"() -> (w808:dbl[])
      }
      frame "time" {
        n613 = local read "Time"() -> (w809:dbl[])
      }
      frame "Lockin1 X" {
        n614 = local read "Lockin1 X"() -> (w810:dbl[])
      }
      frame "Lockin2 X" {
        n615 = local read "Lockin2 X"() -> (w811:dbl[])
      }
      frame "Lockin1 Y" {
        n616 = local read "Lockin1 Y"() -> (w812:dbl[])
      }
      frame "Lockin2 Y" {
        n617 = local read "Lockin2 Y"() -> (w813:dbl[])
      }
      frame "V K2400_01" {
        n618 = local read "V K2400_01 array"() -> (w814:dbl[])
      }
      frame "V K2400_02" {
        n619 = local read "V K2400_02 array"() -> (w815:dbl[])
      }
      frame "I K2400_01" {
        n620 = local read "I K2400 01"() -> (w816:dbl[])
      }
      frame "I K2400_02" {
        n621 = local read "I K2400 02"() -> (w817:dbl[])
      }
      frame "DMM1".."DMM9" {
        n622 = Match Pattern(string=w825, regular expression="DMM") -> (after substring=w823:string)  [unwired: 1 in, 3 out]
        n623 = Scan Value(string=w823, format string="%g") -> (value=w820:dbl)  [unwired: 1 in, 1 out]
        n624 = local read "DMM Array"() -> (w821:dbl[][])
        n625 = Decrement(x=w820) -> (x-1=w818:dbl)
        n626 = Index Array(array=w821, index (col)=w818) -> (element=w819:dbl[])  [unwired: 1 in]
      }
      frame "B" {
        n627 = local read "B"() -> (w826:dbl[])
      }
      frame "R4probe" {
        n628 = local read "R4probe array"() -> (w827:dbl[])
      }
      frame "Formula1" {
        n629 = local read "Formula1Array"() -> (w828:dbl[])
      }
      frame "Formula2" {
        n630 = local read "Formula2Array"() -> (w829:dbl[])
      }
      frame "Formula3" {
        n631 = local read "Formula3Array"() -> (w830:dbl[])
      }
      frame "Formula4" {
        n632 = local read "Formula4Array"() -> (w831:dbl[])
      }
    }
    n633 = call "AxisLabel.vi"("Axis"="X-Axis 4") -> ("X Scale.Name Label.Text"=w551:string)
    n634 = call "AxisLabel.vi"("Axis"="Y-Axis 4") -> ("X Scale.Name Label.Text"=w552:string)
    n635 = property on="Fig 2" class="XYGraph (strict)"("XScale.NameLbl.Text"=w567) -> ()  [unwired: 2 in, 2 out]
    n636 = Decimal String To Number(string="Fig2 Y scale") -> (number=w561:i32)  [unwired: 2 in, 1 out]
    n637 = call "AxisLabel.vi"("Axis"="Y-Axis 2") -> ("X Scale.Name Label.Text"=w568:string)
    n638 = call "AxisLabel.vi"("Axis"="X-Axis 1") -> ("X Scale.Name Label.Text"=w565:string)
    n639 = call "AxisLabel.vi"("Axis"="Y-Axis 1") -> ("X Scale.Name Label.Text"=w564:string)
    n640 = Decimal String To Number(string="Fig1 Y scale") -> (number=w559:i32)  [unwired: 2 in, 1 out]
    n641 = Decimal String To Number(string="Fig3 Y scale") -> (number=w555:i32)  [unwired: 2 in, 1 out]
    n642 = Decimal String To Number(string="Fig3 Y scale 2") -> (number=w550:i32)  [unwired: 2 in, 1 out]
    n643 = property on="Fig 2" class="XYGraph (strict)"("YScale.NameLbl.Text"=w568, "YScale.Mapping Mode"=w561) -> ()  [unwired: 2 in, 2 out]
    n644 = property on="Isd" class="XYGraph (strict)"("XScale.NameLbl.Text"=w565, "YScale.NameLbl.Text"=w564, "YScale.Mapping Mode"=w559) -> ()  [unwired: 2 in, 2 out]
    n645 = property on="Isd 3" class="XYGraph (strict)"("XScale.NameLbl.Text"=w557, "YScale.NameLbl.Text"=w556, "YScale.Mapping Mode"=w555) -> ()  [unwired: 2 in, 2 out]
    n646 = property on="Isd 4" class="XYGraph (strict)"("XScale.NameLbl.Text"=w551, "YScale.NameLbl.Text"=w552, "YScale.Mapping Mode"=w550) -> ()  [unwired: 2 in, 2 out]
    n647 = Quotient & Remainder(x=w533, y=2) -> (floor(x/y)=w531:i32)  [unwired: 1 out]
    n648 = event shown="[3] \"DMMX\": Value Change" {
      selector: _ -> [_ _ _ _]
      dyn-events: _ -> [_ _ _ _]
      timeout: w531 -> [_ _ _ _]
      tunnel: w570 -> [w869 w871 w877 _]
      tunnel: [w869 w871 w877 _] -> w569
      tunnel: w530 -> [_ _ _ w879]
      tunnel: w529 -> [_ _ _ w878]
      event Timeout {
        n649 = event-data() -> ()  [unwired: 1 in, 2 out]
      }
      event "Sensitivity Lockin1": Value Change {
        n650 = event-data() -> ()  [unwired: 1 in, 5 out]
        n651 = local read "Lockin1"() -> (w873:refnum<visa-resource-name>)
        n652 = call "Sr830sens_giulia.vi"("Sr 830 sensitivity"="Sensitivity Lockin1", "Change sensitivity ?"=TRUE, "SR830"=w873) -> ()  [unwired: 1 out]
      }
      event "Sensitivity Lockin2": Value Change {
        n653 = event-data() -> ()  [unwired: 1 in, 5 out]
        n654 = local read "Lockin2"() -> (w875:refnum<visa-resource-name>)
        n655 = call "Sr830sens_giulia.vi"("Sr 830 sensitivity"="Sensitivity Lockin2", "Change sensitivity ?"=TRUE, "SR830"=w875) -> ()  [unwired: 1 out]
      }
      event "DMMX": Value Change {
        n656 = event-data() -> ()  [unwired: 1 in, 5 out]
        n657 = local read "DMMX"() -> (w882:string[][])
        n658 = Array Size(array=w882) -> (size(s)=w881:i32[])
        n659 = Index Array(array=w881, index=0) -> (element=w883:i32)
        n660 = for {
          N: w883 -> [_]
          tunnel: w882 -> [_] mode=indexing
          tunnel: [w887] -> w885 mode=indexing
          i -> [w890]
          n661 = Increment(x=w890) -> (x+1=w888:i32)
          n662 = Number To Decimal String(number=w888) -> (decimal integer string=w889:string)  [unwired: 1 in]
          n663 = Concatenate Strings("DMM", w889) -> (w887:string)
        }
        n664 = Insert Into Array(array=w878, new element=w885) -> (w886:string[])  [unwired: 1 in]
        n665 = Insert Into Array(array=w879, new element=w885) -> (w884:string[])  [unwired: 1 in]
        n666 = property on="Vsd" class="CmbBox"("Strings[]"=w886) -> ()  [unwired: 2 in, 2 out]
        n667 = property on="I leak BG" class="CmbBox"("Strings[]"=w886) -> ()  [unwired: 2 in, 2 out]
        n668 = property on="I leak TG" class="CmbBox"("Strings[]"=w886) -> ()  [unwired: 2 in, 2 out]
        n669 = property on="Vxx" class="CmbBox"("Strings[]"=w886) -> ()  [unwired: 2 in, 2 out]
        n670 = property on="I 2probe 2" class="CmbBox"("Strings[]"=w886) -> ()  [unwired: 2 in, 2 out]
        n671 = property on="Vxy" class="CmbBox"("Strings[]"=w886) -> ()  [unwired: 2 in, 2 out]
        n672 = property on="V TG" class="CmbBox"("Strings[]"=w886) -> ()  [unwired: 2 in, 2 out]
        n673 = property on="V BG" class="CmbBox"("Strings[]"=w886) -> ()  [unwired: 2 in, 2 out]
        n674 = property on="Y-Axis 4" class="CmbBox"("Strings[]"=w884) -> ()  [unwired: 2 in, 2 out]
        n675 = property on="X-Axis 4" class="CmbBox"("Strings[]"=w884) -> ()  [unwired: 2 in, 2 out]
        n676 = property on="Y-Axis 1" class="CmbBox"("Strings[]"=w884) -> ()  [unwired: 2 in, 2 out]
        n677 = property on="X-Axis 1" class="CmbBox"("Strings[]"=w884) -> ()  [unwired: 2 in, 2 out]
        n678 = property on="X-Axis 2" class="CmbBox"("Strings[]"=w884) -> ()  [unwired: 2 in, 2 out]
        n679 = property on="Y-Axis 2" class="CmbBox"("Strings[]"=w884) -> ()  [unwired: 2 in, 2 out]
        n680 = property on="X-Axis 3" class="CmbBox"("Strings[]"=w884) -> ()  [unwired: 2 in, 2 out]
        n681 = property on="Y-Axis 3" class="CmbBox"("Strings[]"=w884) -> ()  [unwired: 2 in, 2 out]
      }
    }
    n682 = Bundle("Formula4Array"=w540, "Formula4Array"=w539) -> (→"Fig 2":T10)  [unwired: 1 out]
    n683 = Bundle("Formula4Array"=w537, "Formula4Array"=w535) -> (→"Isd":T10)  [unwired: 1 out]
    n684 = Bundle("Formula4Array"=w543, "Formula4Array"=w545) -> (→"Isd 3":T10)  [unwired: 1 out]
    n685 = Bundle("Formula4Array"=w549, "Formula4Array"=w547) -> (→"Isd 4":T10)  [unwired: 1 out]
  }
  n686 = Insert Into Array(array=w2, new element=w4) -> (w5:string[])  [unwired: 1 in]
  n687 = Insert Into Array(array=w1, new element=w4) -> (w3:string[])  [unwired: 1 in]
  n688 = property on="Y-Axis 4" class="CmbBox"("Strings[]"=w5) -> ()  [unwired: 2 in, 2 out]
  n689 = property on="X-Axis 4" class="CmbBox"("Strings[]"=w5) -> ()  [unwired: 2 in, 2 out]
  n690 = property on="Y-Axis 1" class="CmbBox"("Strings[]"=w5) -> ()  [unwired: 2 in, 2 out]
  n691 = property on="X-Axis 1" class="CmbBox"("Strings[]"=w5) -> ()  [unwired: 2 in, 2 out]
  n692 = property on="X-Axis 2" class="CmbBox"("Strings[]"=w5) -> ()  [unwired: 2 in, 2 out]
  n693 = property on="Y-Axis 2" class="CmbBox"("Strings[]"=w5) -> ()  [unwired: 2 in, 2 out]
  n694 = property on="X-Axis 3" class="CmbBox"("Strings[]"=w5) -> ()  [unwired: 2 in, 2 out]
  n695 = property on="Y-Axis 3" class="CmbBox"("Strings[]"=w5) -> ()  [unwired: 2 in, 2 out]
  n696 = property on="Vsd" class="CmbBox"("Strings[]"=w3) -> ()  [unwired: 2 in, 2 out]
  n697 = property on="I leak BG" class="CmbBox"("Strings[]"=w3) -> ()  [unwired: 2 in, 2 out]
  n698 = property on="I leak TG" class="CmbBox"("Strings[]"=w3) -> ()  [unwired: 2 in, 2 out]
  n699 = property on="Vxx" class="CmbBox"("Strings[]"=w3) -> ()  [unwired: 2 in, 2 out]
  n700 = property on="I 2probe 2" class="CmbBox"("Strings[]"=w3) -> ()  [unwired: 2 in, 2 out]
  n701 = property on="Vxy" class="CmbBox"("Strings[]"=w3) -> ()  [unwired: 2 in, 2 out]
  n702 = property on="V TG" class="CmbBox"("Strings[]"=w3) -> ()  [unwired: 2 in, 2 out]
  n703 = property on="V BG" class="CmbBox"("Strings[]"=w3) -> ()  [unwired: 2 in, 2 out]
